vi "CSM - Debug Console - previous.vi"() -> ()   [LabVIEW 2017]
doc: "CSM Debug Console, you can use this tool:\n\n1. Select an existing CSM instance, open the front panel and block diagram.\n2. Scan the API interfaces of existing CSM instances.\n3. Select an API interface, call synchronously or asynchronously, view the return value.\n4. View the overall program's running log."
uses:
  _Support/Typedef/_CSM_List Module Scope.ctl
  Utility/_support/Periodic String Filter Level.ctl
  Utility/Periodic String Filter Setting.ctl
  _Support/Typedef/_CSM_GlobalLog_MSG.ctl
  _Support/Typedef/_CSM_Response Source Message.ctl
  _Support/Typedef/_CSM_GlobalLog_MSG_TYPE.ctl
  1437127e-efa5-494e-aa43-da9d647a7a6f.vi
  6c6a0a0d-4e90-432b-9646-7a8ac0ceadb8.vi
  AdvanceAPI/CSM - Keywords.vi
  AdvanceAPI/CSM - Convert Error to Argument.vi
  _Support/GlobalEvent/GEvt-Generate with Rule Check.vi
  _Support/GlobalEvent/Cache-GEvt Refs.vi
  _Shared/Change Speed Counter.vi
  _Support/ChangeFlag/FlagInstance-GEvt Refs.vi
  _Support/ChangeFlag/ChangeFlag-Read.vi
  _Support/GlobalEvent/LogFilter/LogFilter - Check.vi
  _Support/GlobalEvent/GEvt-Valid Subscribers.vi
  _Support/GlobalEvent/FGV-GlobalEventQueues(lvlibp).vi
  _Support/GlobalEvent/FGV-GlobalEventRef(lvlibp).vi
  _Support/ChangeFlag/ChangeFlagDB.vi
  _Polymophic/Build Interrupt Broadcast Message.vi
  _Polymophic/Build No-Reply Asynchronous Message with Arguments.vi
  _Polymophic/Build Synchronous Message with Arguments.vi
  <vilib>/Utility/config.llb/Close Config Data.vi
  <vilib>/Utility/config.llb/Write Key.vi
  <vilib>/Utility/config.llb/Write Key (Double).vi
  <vilib>/Utility/config.llb/Write Key (I32).vi
  <vilib>/Utility/config.llb/Write Key (String).vi
  _csmHelper/lvcsmFile/Path to lvcsm String.vi
  <vilib>/Utility/config.llb/Remove Key.vi
  <vilib>/Utility/config.llb/Get Key Names.vi
  <vilib>/Utility/Data Type/Get Type Information.vi
  <vilib>/Utility/Data Type/Get Array Information.vi
  <vilib>/Utility/config.llb/Write Key (Boolean).vi
  <vilib>/Utility/config.llb/Open Config Data.vi
  _csmHelper/lvcsmFile/lvcsm File Path.vi
  _csmHelper/lvcsmFile/_Array of VData to VCluster.vi
  <vilib>/Utility/config.llb/Read Key.vi
  <vilib>/Utility/config.llb/Read Key (Double).vi
  <vilib>/Utility/config.llb/Read Key (I32).vi
  _csmHelper/lvcsmFile/lvcsm String to Path.vi
  <vilib>/Utility/config.llb/Read Key (String).vi
  <vilib>/Utility/config.llb/Read Key (Boolean).vi
  _Polymophic/Add State(s) to Queue By BOOL(Element).vi
  _csmHelper/API/Destroy.vi
  _csmHelper/API/Update lvcsm Section in VI Description.vi
  _csmHelper/API/Create From VI Reference.vi
  _Support/GlobalEvent/LogFilter/LogFilter.lvclass
  Communicable State Machine.lvlib
  _csmHelper/API with lvcsm Support/CSM-Helper API with lvcsm Support.lvlib
  _csmHelper/CSM-Helper.lvclass
  _Support/csm-tool-support.lvlib
  _Shared/CSM Shared.lvlib
  _ui/csm-ui-support.lvlib
panel:
  in  "Scope":T1
  in  "Refresh CSMs Button":bool
  in  "CSM":string(combo)
  in  "Write lvcsm in Description":bool
  out "inlvlibp":bool
  in  "RetainWireValues":bool
  in  "Interface-Filter":enum16{"API-Only", "UserDef States", "All"}(ring)
  in  "Toolbar.Exit":bool
  in  "Toolbar.Open FP":bool
  in  "Toolbar.Open BD":bool
  in  "Refresh lvcsm Cache":bool
  in  "History":i32(listbox)
  in  "Refresh API":bool
  in  "MsgString":string(combo)
  in  "Tab(Msg/Status)":enum32{"Message", "Status"}(tab)
  in  "Sync (-@)":bool
  in  "Async (->|)":bool
  in  "Timeout(s)":i32=10 caption="(s)" min=1 max=180 step=1 format="%.0p"
  in  "Broadcast":bool
  in  "Arguments":string
  in  "Revert Safe String":bool=TRUE
  out "Response":string
  in  "Periodic":bool
  in  "Settings":T2={"threashold(#/s)"=0.5, "Check Peroid(s)"=3.0}
  in  "Periodic Info":bool=TRUE
  in  "internal-stop":bool
  out "handling Speed(#/s)":dbl
  in  "Level":T3
  out "LogInQ":i32
  out "State History":string
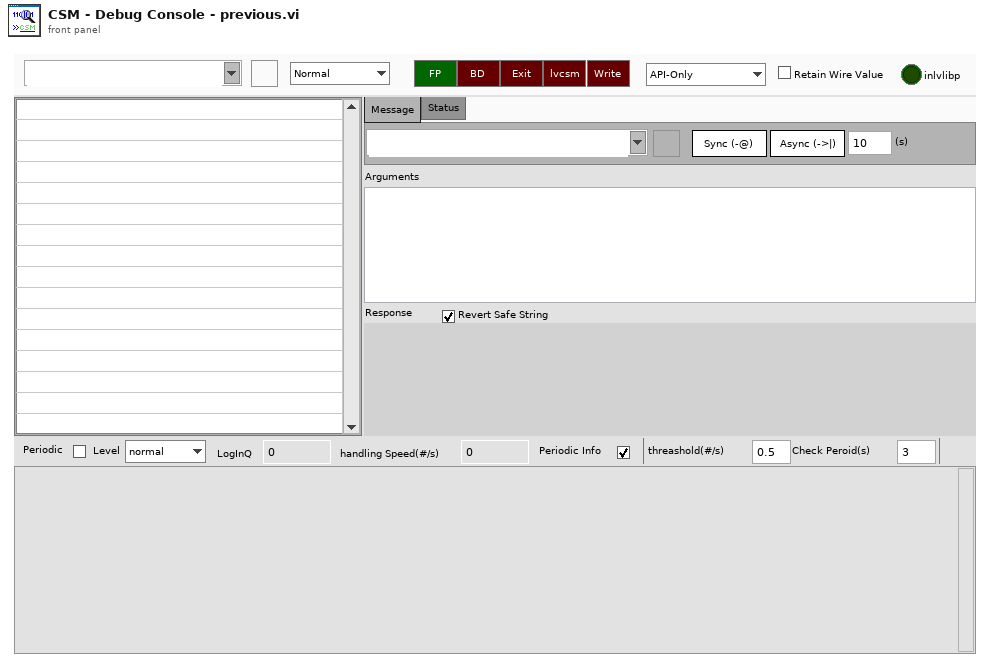
[diagram p1: front panel]
types:
  T1 = typedef "Communicable State Machine.lvlib/_CSM_List Module Scope.ctl" = enum16{"Normal", "System Only", "All"}
  T2 = typedef "Communicable State Machine.lvlib/Periodic String Filter Setting.ctl" = cluster{"threashold(#/s)":dbl, "Check Peroid(s)":dbl}
  T3 = typedef "Communicable State Machine.lvlib/Periodic String Filter Level.ctl" = enum16{"normal", "L1", "L2", "L3", "L4"}
  T4 = enum32{"Invalid", "Standard", "Closed", "Hidden", "Minimized", "Maximized"}
  T5 = enum32{"invalid app kind", "Development System", "Run Time System", "Student Edition", "Embedded LabVIEW", "Evaluation", "Custom"}
  T6 = cluster{"Response Timeout(s)":i32, "History Length":i32, "History":string[], "Periodic Enable":bool, "Periodic threashold(#/s)":dbl, "Periodic Check Peroid(s)":dbl}
  T7 = enum8{"Enabled", "Disabled", "Disabled and Grayed Out"}
  T8 = cluster{"Shift":bool, "Ctrl":bool, "Alt":bool, "Cmd":bool, "Opt":bool}
  T9 = typedef "LVPoint32TypeDef.ctl" = cluster{"Horizontal":i32, "Vertical":i32}
  T10 = cluster{"Core":cluster{"Current VI Reference":refnum<vi>, "Close Panel on Exit?":bool}, "CSM Global Log Event":refnum<user-event>, "MessageList":string[], "Toobar.advance":refnum<vi>[], "CSM Check History":string[], "History Length":i32}
  T11 = cluster{"Current VI Reference":refnum<vi>, "Close Panel on Exit?":bool}
  T12 = cluster{"Periodic threashold(#/s)":dbl, "Periodic Check Peroid(s)":dbl}
  T13 = typedef "Communicable State Machine.lvlib/_CSM_GlobalLog_MSG.ctl" = cluster{"Name (\"\" to Use UUID)":string, "Current State":string, "Arguments":string, "Source Message":T14, "Source Module":string, "Complete(T)/Start(F)":bool, "LogType":T15, "Time Stamp":timestamp}
  T14 = typedef "Communicable State Machine.lvlib/_CSM_Response Source Message.ctl" = cluster{"‘State":string, "’Arguments":string, "’Error":errorcluster}
  T15 = typedef "Communicable State Machine.lvlib/_CSM_GlobalLog_MSG_TYPE.ctl" = enum16{"User Log", "State Change", "Status", "Interrupt", "Register", "Unregister", "Error Log", "Module Created", "Module Destroyed", "Async Message", "No-Rep Async Message", "Sync Message"}
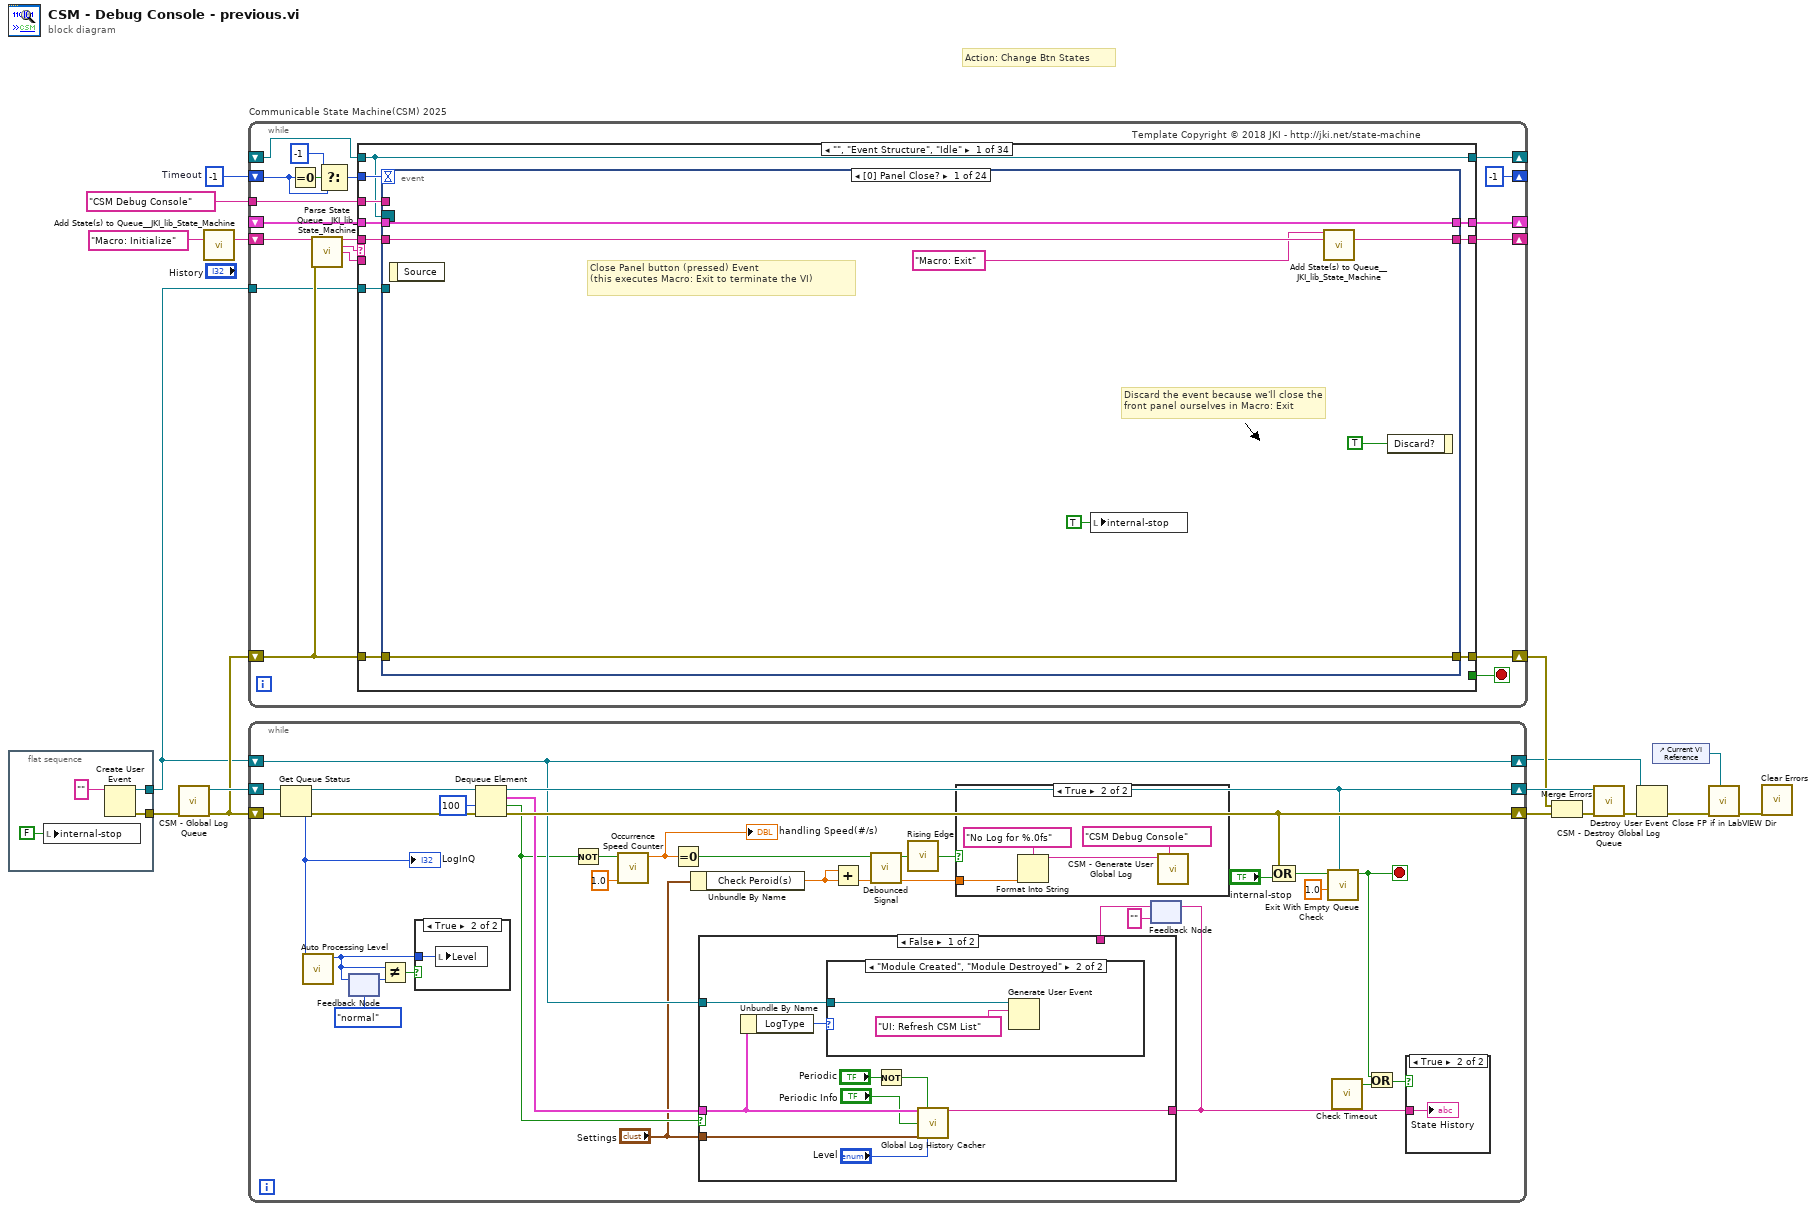
[diagram p0: block diagram]
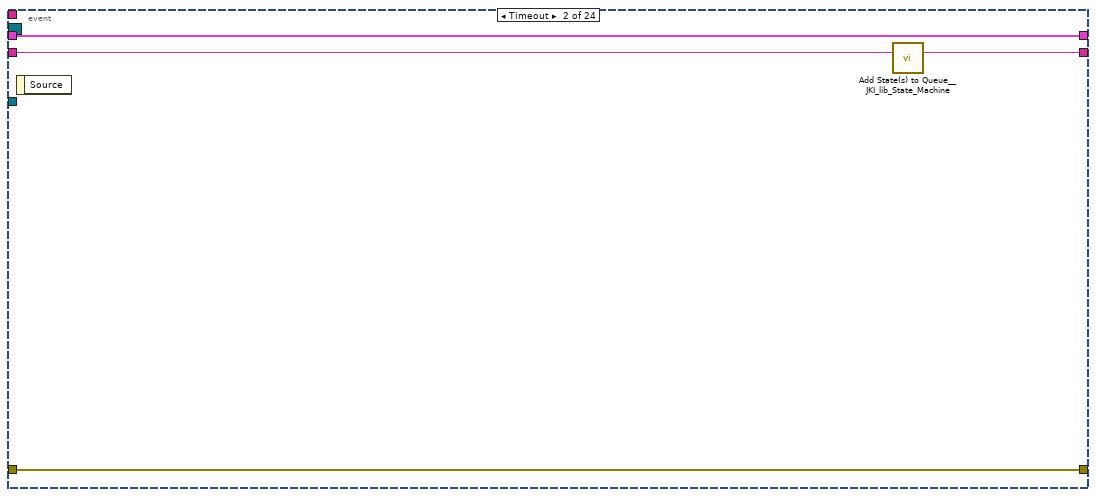
[diagram p7: hidden frame]
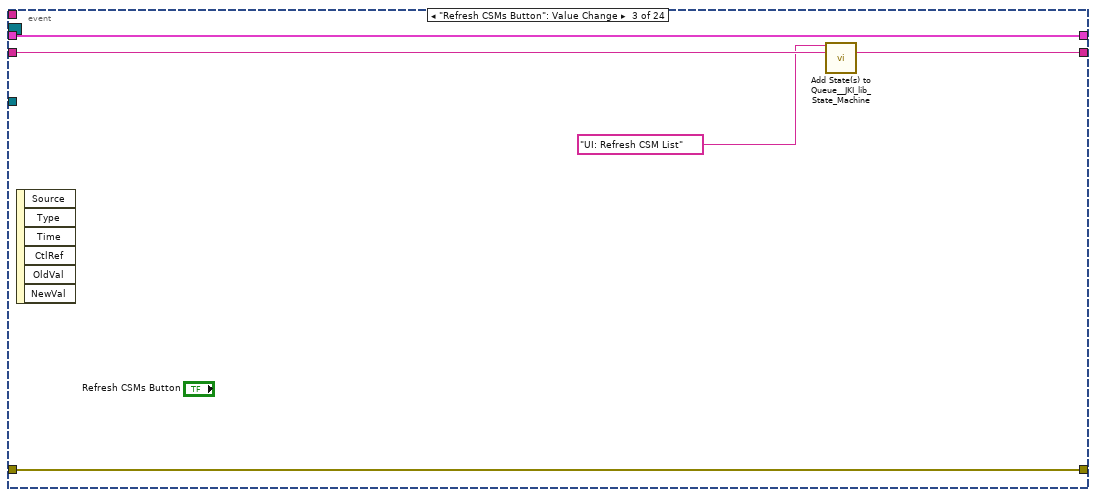
[diagram p8: hidden frame]
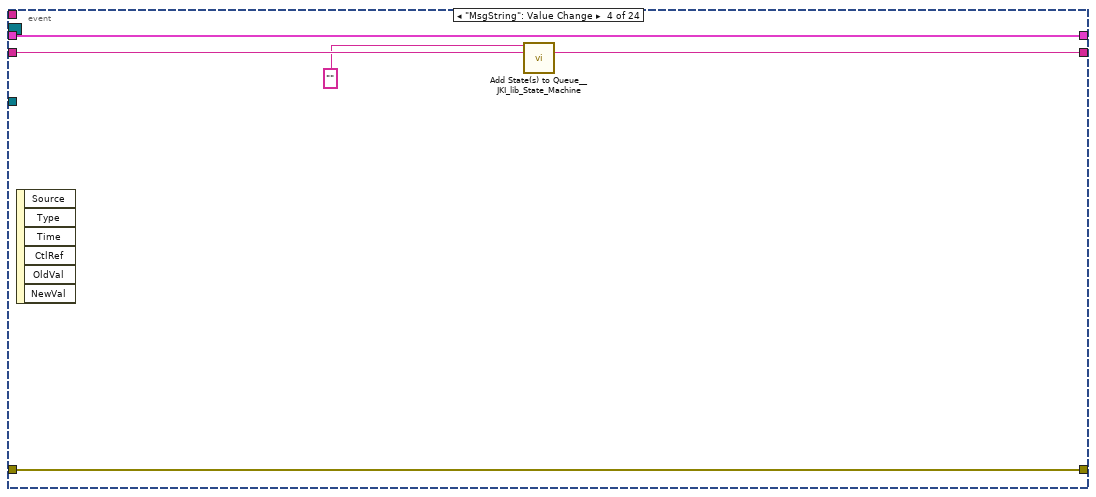
[diagram p9: hidden frame]
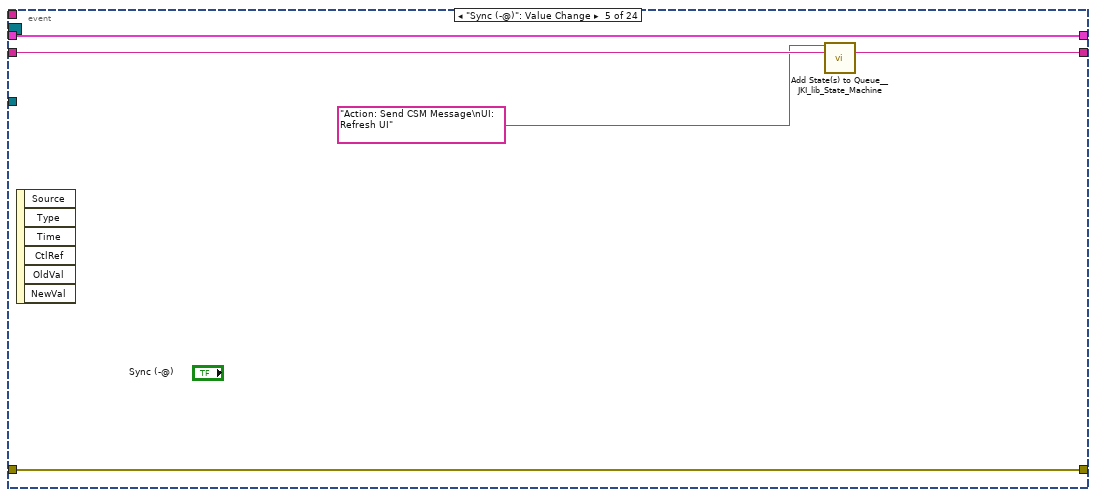
[diagram p10: hidden frame]
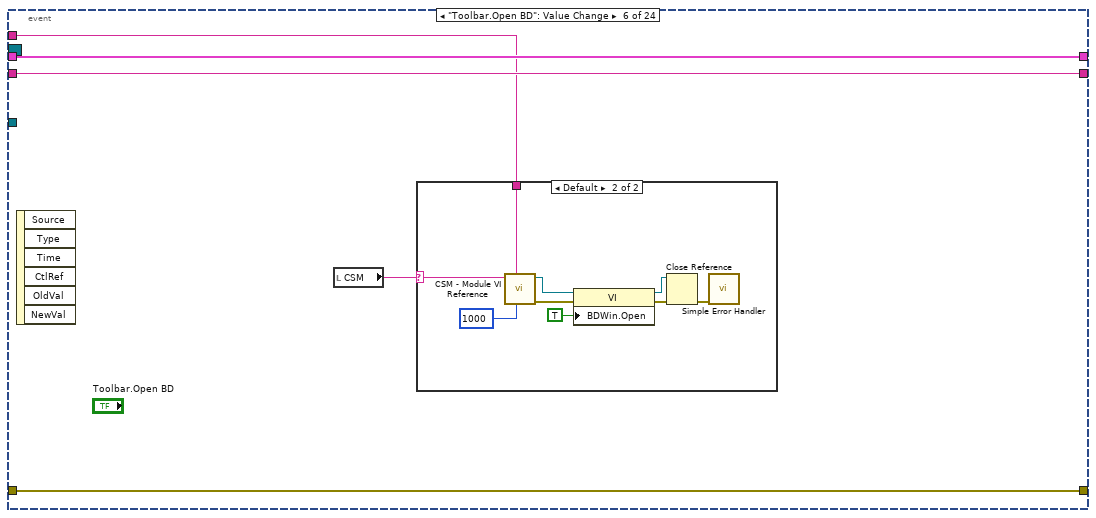
[diagram p11: hidden frame]
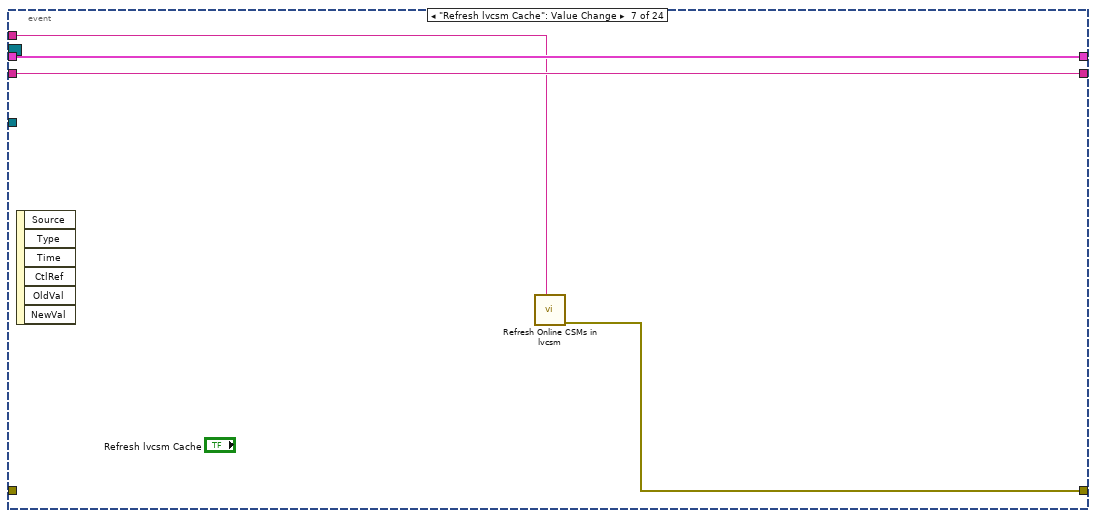
[diagram p13: hidden frame]
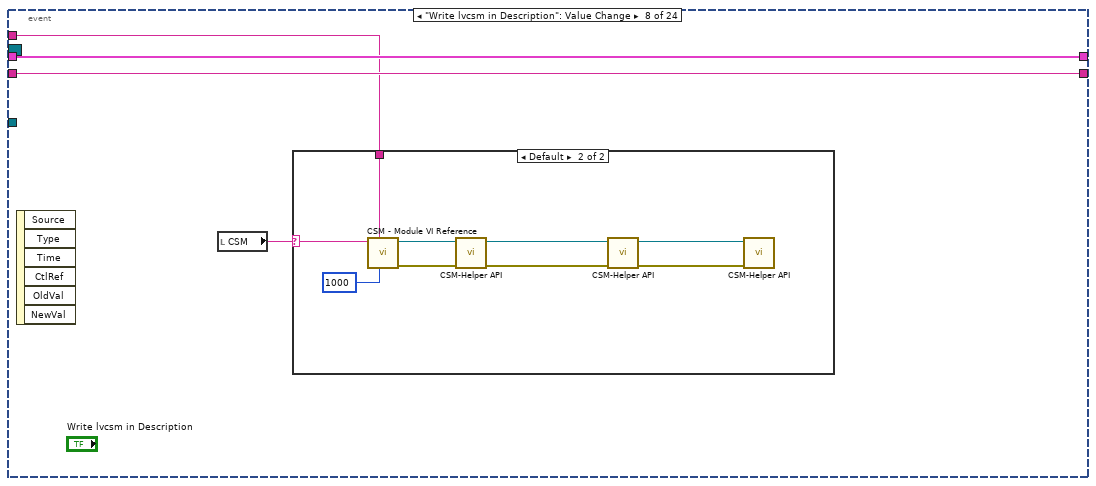
[diagram p14: hidden frame]
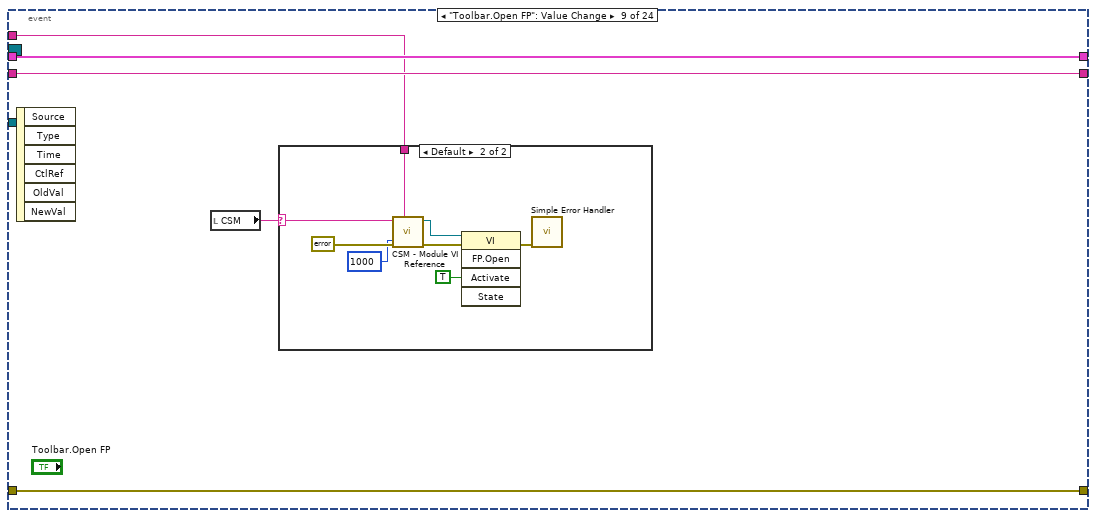
[diagram p16: hidden frame]
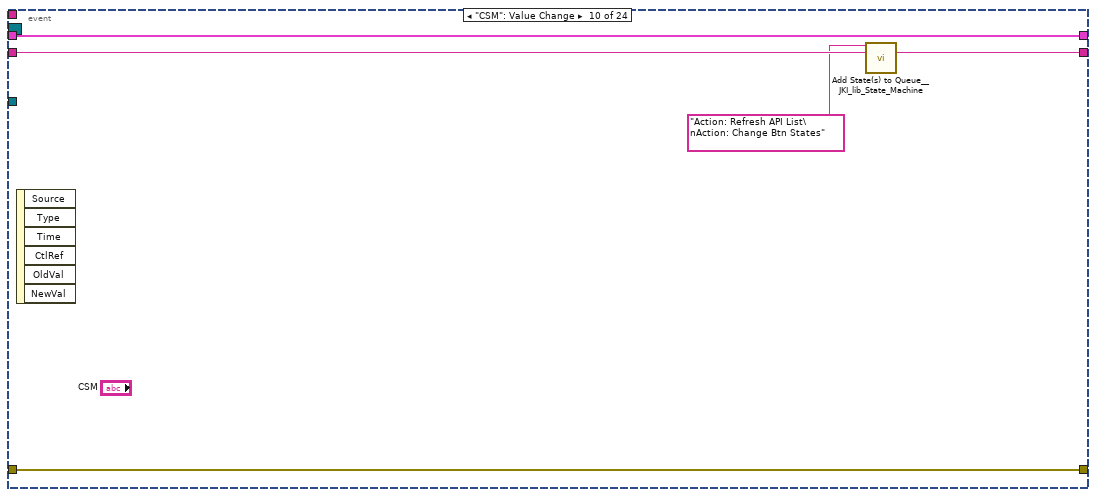
[diagram p18: hidden frame]
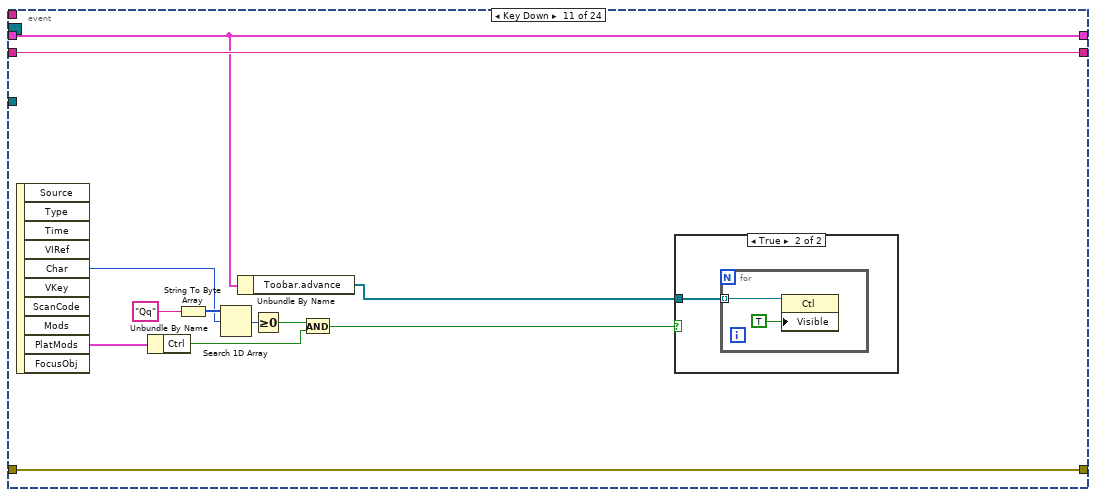
[diagram p19: hidden frame]
diagram:
  w14 = -1  # Timeout
  # "Action: Change Btn States"
  n1 = flat-sequence {
    tunnel: [w21] -> w7
    tunnel: [w19] -> w4
    frame #0 {
      n2 = local write "internal-stop"(FALSE ("internal-stop")) -> ()
      n3 = Create User Event(user event datatype="" ("UserEvent")) -> (user event=w19:refnum<user-event>, error out=w21:errorcluster)  [unwired: 1 in]
    }
  }
  n4 = call "CSM - Global Log Queue.vi"("Error In"=w7) -> ("error out"=w10:errorcluster, "Global Log Queue"=w11:refnum<queue>)  [unwired: 9 in]
  n5 = call <vilib>:"Add State(s) to Queue__JKI_lib_State_Machine.vi"("State(s) in (\"\")"="Macro: Initialize") -> ("States Out"=w16:string)  [unwired: 14 in]
  n6 = while "Communicable State Machine(CSM) 2025" {
    shift-right: [w33] -> _
    shift-left: _ -> [w32]
    shift-right: [w36] -> w8
    shift-left: w10 -> [w31]
    shift-right: [w35] -> _
    shift-left: w16 -> [w37]
    tunnel: "CSM Debug Console" -> [w30]
    shift-right: [-1 ("Timeout")] -> _
    shift-left: w14 -> [w27]
    tunnel: w4 -> [w24]
    shift-right: [w23] -> _
    shift-left: _ -> [w22]
    stop <- w34 stop-if-true
    # "Template Copyright © 2018 JKI - http://jki.net/state-machine"
    n7 = Equal To 0?(x=w27) -> (x = 0?=w29:bool)
    n8 = call <vilib>:"Parse State Queue__JKI_lib_State_Machine.vi"("State Queue"=w37, "Error In (no error)"=w31) -> ("Remaining States"=w39:string, "Current State"=w40:string, "Arguments"=w38:string)  [unwired: 11 in]
    n9 = Select(t=-1 ("Timeout"), s=w29, f=w27) -> (s? t:f=w26:i32)
    n10 = case shown="\"\", \"Event Structure\", \"Idle\"" w40 {
      selector: w40 -> [_ _ w312 _ _ _ _ _ _ _ _ _ _ _ _ _ _ _ _ _ _ _ _ _ _ _ _ _ _ _ _ _ _ _]
      tunnel: w39 -> [w50 w310 w316 w336 w344 w350 w355 w366 w374 w389 w403 w416 w432 w437 w442 w447 w452 w462 w472 w484 w564 w581 w595 w599 w605 w611 w622 w627 w639 w666 w686 w703 w733 w789]
      tunnel: w38 -> [_ _ _ _ _ _ _ _ _ _ _ w412 _ _ _ _ _ _ w467 w478 w563 _ _ _ _ _ _ _ _ _ _ _ _ _]
      tunnel: w32 -> [w48 w307 w314 w329 w341 w348 w352 _ w373 w387 w402 w414 w427 w434 w440 w445 w449 w459 w470 w480 w561 w580 w594 w598 w602 w608 w619 w624 w637 w664 w684 w702 w728 w788]
      tunnel: [w47 w308 w318 w333 errorcluster {"status"=FALSE, "code"=0, "source"=""} ("error out") w347 w353 w363 w375 _ w397 w415 w428 w435 _ w443 w450 w460 w468 w481 w565 w582 w596 w600 w603 w609 w620 w625 w634 w663 w683 w704 w730 w790] -> w36
      tunnel: w31 -> [w46 w308 w317 w333 w340 w347 w353 w363 w375 _ _ w415 w429 w435 _ _ w450 w460 w469 w482 w565 w582 w596 w600 w603 w609 w620 w625 _ _ _ w704 _ w790]
      tunnel: [w49 w309 w315 w335 w343 w349 w354 w365 w374 w389 w403 w416 w431 w436 w441 w446 w451 w461 w471 w483 w564 w581 w595 w599 w604 w610 w621 w626 w638 w665 w685 w703 w733 w789] -> w35
      tunnel: [_ _ _ _ _ TRUE _ _ _ _ _ _ _ _ _ _ _ _ _ _ _ _ _ _ _ _ _ _ _ _ _ _ _ _] -> w34
      tunnel: [w45 w307 w314 w334 w341 w348 w352 w364 w370 w388 w402 w408 w427 w434 w440 w445 w449 w459 w470 w480 w561 w580 w594 w598 w602 w608 w619 w624 w637 w664 w684 w702 w727 w788] -> w33
      tunnel: w26 -> [w44 _ _ _ _ _ _ _ _ _ _ _ _ _ _ _ _ _ _ _ _ _ _ _ _ _ _ _ _ _ _ _ _ _]
      tunnel: w30 -> [w43 _ _ _ w338 _ _ _ _ w384 w398 _ _ _ _ _ _ _ _ _ _ _ _ _ _ _ _ _ _ _ _ w699 w731 w785]
      tunnel: w24 -> [w42 _ _ _ _ _ _ _ _ _ _ _ _ _ w439 _ _ _ _ _ _ _ _ _ _ _ _ _ _ _ _ _ _ _]
      tunnel: [w41 w306 w311 w323 w337 w345 w351 w357 w367 w382 w396 w405 w426 w433 w438 w444 w448 w455 w466 w477 w553 w576 w583 w597 w601 w606 w612 w623 w628 w658 w678 w701 w725 w787] -> w23
      tunnel: w22 -> [w41 w306 w311 w323 w337 w345 w351 w357 w367 w382 w396 w405 w426 w433 _ w444 w448 w455 w466 w477 w553 w576 w583 w597 w601 w606 w612 w623 w628 w658 w678 w701 w725 w787]
      frame "", "Event Structure", "Idle" {
        n11 = event shown="[0] Panel Close?" {
          selector: w41 -> [_ _ _ _ _ _ _ _ _ _ _ _ _ _ _ _ _ _ _ _ _ _ _ _]
          dyn-events: _ -> [_ _ _ _ _ _ _ _ _ _ _ _ _ _ _ _ _ _ _ _ _ _ _ _]
          timeout: w44 -> [_ _ _ _ _ _ _ _ _ _ _ _ _ _ _ _ _ _ _ _ _ _ _ _]
          tunnel: w50 -> [w57 w61 w64 w68 w73 w81 w94 w98 w112 w122 w137 w142 w148 w156 w166 w173 w201 w220 w239 w252 w257 w262 w274 w276]
          tunnel: [w56 w60 w63 w69 w74 w81 w94 w98 w112 w123 w137 w143 w148 w157 w167 w173 w201 w220 w239 w253 w258 w263 w274 w278] -> w49
          tunnel: w48 -> [w54 w58 w65 w70 w75 w80 w93 w97 w111 w124 w126 w144 w146 w163 w168 w172 w199 w218 w237 w254 w259 w264 w272 w279]
          tunnel: [w55 w59 w66 w71 w76 w78 w91 _ w109 w125 w136 w145 w147 w164 _ w171 w200 w219 w238 w255 w260 _ w273 w280] -> w47
          tunnel: w46 -> [w55 w59 w66 w71 w76 w78 _ _ w109 w125 w136 w145 w147 w164 _ w171 w200 w219 w238 w255 w260 _ w273 w280]
          tunnel: [w54 w58 w65 w70 w75 w80 w93 w97 w111 w124 w126 w144 w146 w163 w168 w172 w199 w218 w237 w254 w259 w264 w272 w277] -> w45
          tunnel: w43 -> [_ _ _ _ _ w77 w92 w95 w108 _ _ _ _ _ _ w169 _ w216 _ _ _ _ _ _]
          tunnel: w42 -> [_ _ _ _ _ _ _ _ _ _ _ _ _ _ _ _ _ _ _ _ _ _ _ _]
          event Panel Close? {
            # "Discard the event because we'll close the front panel ourselves in Macro: Exit"
            # "Close Panel button (pressed) Event\n(this executes Macro: Exit to terminate the VI)"
            n12 = event-data() -> ()  [unwired: 1 in, 1 out]
            n13 = local write "internal-stop"(TRUE ("internal-stop")) -> ()
            n14 = call <vilib>:"Add State(s) to Queue__JKI_lib_State_Machine.vi"("State(s) in Front (\"\")"="Macro: Exit", "State(s) in (\"\")"=w57) -> ("States Out"=w56:string)  [unwired: 13 in]
            n15 = event-data("Discard?"=TRUE) -> ()  [unwired: 1 in, 1 out]
          }
          event Timeout {
            n16 = event-data() -> ()  [unwired: 1 in, 1 out]
            n17 = call <vilib>:"Add State(s) to Queue__JKI_lib_State_Machine.vi"("State(s) in (\"\")"=w61) -> ("States Out"=w60:string)  [unwired: 14 in]
          }
          event "Refresh CSMs Button": Value Change {
            n18 = event-data() -> ()  [unwired: 1 in, 6 out]
            n19 = call <vilib>:"Add State(s) to Queue__JKI_lib_State_Machine.vi"("State(s) in Front (\"\")"="UI: Refresh CSM List" ("State(s) in Front (\"\")"), "State(s) in (\"\")"=w64) -> ("States Out"=w63:string)  [unwired: 13 in]
          }
          event "MsgString": Value Change {
            n20 = event-data() -> ()  [unwired: 1 in, 6 out]
            n21 = call <vilib>:"Add State(s) to Queue__JKI_lib_State_Machine.vi"("State(s) in Front (\"\")"="" ("State(s) in Front (\"\")"), "State(s) in (\"\")"=w68) -> ("States Out"=w69:string)  [unwired: 13 in]
          }
          event "Sync (-@)": Value Change {
            n22 = event-data() -> ()  [unwired: 1 in, 6 out]
            n23 = call <vilib>:"Add State(s) to Queue__JKI_lib_State_Machine.vi"("State(s) in Front (\"\")"="Action: Send CSM Message\nUI: Refresh UI" ("State(s) in Front (\"\")"), "State(s) in (\"\")"=w73) -> ("States Out"=w74:string)  [unwired: 13 in]
          }
          event "Toolbar.Open BD": Value Change {
            n24 = event-data() -> ()  [unwired: 1 in, 6 out]
            n25 = local read "CSM"() -> (w79:string)
            n26 = case shown="Default" w79 {
              selector: w79 -> [_ w89]
              tunnel: w77 -> [_ w88]
              frame "" {
              }
              frame Default {
                n27 = call "CSM - Module VI Reference.vi"("Response Timeout (-2 Using Global Settings)"=1000 ("Response Timeout(5000 ms)"), "Current Module (\"\" to Generate an ID)"=w88, "CSM Name"=w89) -> ("error out"=w82:errorcluster, "CSM Module VIRef"=w87:refnum<vi>)  [unwired: 7 in]
                n28 = property class="VI"(reference=w87, error in=w82, "BDWin.Open"=TRUE ("Block Diagram Window:Open")) -> (reference out=w85:refnum<vi>, error out=w84:errorcluster)
                n29 = Close Reference(reference=w85, error in (no error)=w84) -> (error out=w90:errorcluster)
                n30 = call <vilib>:"Simple Error Handler.vi"("error in (no error)"=w90) -> ()  [unwired: 4 in, 5 out]
              }
            }
          }
          event "Refresh lvcsm Cache": Value Change {
            n31 = event-data() -> ()  [unwired: 1 in, 6 out]
            n32 = call "Refresh Online CSMs in lvcsm.vi"("Caller"=w92) -> ("error out"=w91:errorcluster)  [unwired: 9 in, 1 out]
          }
          event "Write lvcsm in Description": Value Change {
            n33 = event-data() -> ()  [unwired: 1 in, 6 out]
            n34 = local read "CSM"() -> (w96:string)
            n35 = case shown="Default" w96 {
              selector: w96 -> [_ w103]
              tunnel: w95 -> [_ w99]
              frame "" {
              }
              frame Default {
                n36 = call "CSM - Module VI Reference.vi"("Response Timeout (-2 Using Global Settings)"=1000 ("Response Timeout(5000 ms)"), "Current Module (\"\" to Generate an ID)"=w99, "CSM Name"=w103) -> ("error out"=w101:errorcluster, "CSM Module VIRef"=w100:refnum<vi>)  [unwired: 7 in]
                n37 = call-poly "CSM-Helper API.vi"("error in (no error)"=w101, "VI"=w100) -> ("error out"=w107:errorcluster, "CSM-Helper.lvclass"=w106:refnum<class "CSM-Helper.lvclass">)  [unwired: 8 in]
                n38 = call-poly "CSM-Helper API.vi"("error in (no error)"=w107, "CSM-Helper in"=w106) -> ("error out"=w105:errorcluster, "CSM-Helper out"=w104:refnum<class "CSM-Helper.lvclass">)  [unwired: 8 in]
                n39 = call-poly "CSM-Helper API.vi"("error in (no error)"=w105, "CSM-Helper in"=w104) -> ()  [unwired: 8 in, 2 out]
              }
            }
          }
          event "Toolbar.Open FP": Value Change {
            n40 = event-data() -> ()  [unwired: 1 in, 6 out]
            n41 = local read "CSM"() -> (w110:string)
            n42 = case shown="Default" w110 {
              selector: w110 -> [_ w120]
              tunnel: w108 -> [_ w118]
              frame "" {
              }
              frame Default {
                n43 = call "CSM - Module VI Reference.vi"("Response Timeout (-2 Using Global Settings)"=1000 ("Response Timeout(5000 ms)"), "Current Module (\"\" to Generate an ID)"=w118, "error in (no error)"=errorcluster {"status"=FALSE, "code"=0, "source"=""}, "CSM Name"=w120) -> ("error out"=w114:errorcluster, "CSM Module VIRef"=w115:refnum<vi>)  [unwired: 6 in]
                n44 = invoke on="Invoke Node" class="VI" method="FP.Open"(reference=w115, error in=w114, "Activate"=TRUE ("Activate?")) -> (error out=w119:errorcluster)  [unwired: 2 in, 4 out]
                n45 = call <vilib>:"Simple Error Handler.vi"("error in (no error)"=w119) -> ()  [unwired: 4 in, 5 out]
              }
            }
          }
          event "CSM": Value Change {
            n46 = event-data() -> ()  [unwired: 1 in, 6 out]
            n47 = call <vilib>:"Add State(s) to Queue__JKI_lib_State_Machine.vi"("State(s) in Front (\"\")"="Action: Refresh API List\nAction: Change Btn States" ("State(s) in Front (\"\")"), "State(s) in (\"\")"=w122) -> ("States Out"=w123:string)  [unwired: 13 in]
          }
          event Key Down {
            n48 = event-data() -> ("Char"=w127:i16, "PlatMods"=w128:T8)  [unwired: 1 in, 8 out]
            n49 = Unbundle By Name(w128) -> ("Ctrl"=w131:bool)
            n50 = String To Byte Array(string="Qq") -> (unsigned byte array=w133:u8[])
            n51 = Search 1D Array(1D array=w133, element=w127) -> (index of element=w134:i32)  [unwired: 1 in]
            n52 = Unbundle By Name(w126) -> ("Toobar.advance"=w129:refnum<vi>[])
            n53 = Greater Or Equal To 0?(x=w134) -> (x >= 0?=w135:bool)
            n54 = And(x=w135, y=w131) -> (x .and. y?=w130:bool)
            n55 = case shown="True" w130 {
              tunnel: w129 -> [_ w138]
              frame False {
              }
              frame True {
                n56 = for {
                  tunnel: w138 -> [w140] mode=indexing
                  n57 = property class="Ctl"(reference=w140, "Visible"=TRUE) -> ()  [unwired: 1 in, 2 out]
                }
              }
            }
          }
          event "Async (->|)": Value Change {
            n58 = event-data() -> ()  [unwired: 1 in, 6 out]
            n59 = call <vilib>:"Add State(s) to Queue__JKI_lib_State_Machine.vi"("State(s) in Front (\"\")"="Action: Post CSM Message" ("State(s) in Front (\"\")"), "State(s) in (\"\")"=w142) -> ("States Out"=w143:string)  [unwired: 13 in]
          }
          event "Timeout(s)": Value Change {
            n60 = event-data() -> ()  [unwired: 1 in, 6 out]
          }
          event "History": Double Click {
            n61 = event-data() -> ("CtlRef"=w162:refnum<vi>, "Coords"=w150:T9)  [unwired: 1 in]
            n62 = invoke class="LstBox (strict)" method="Point To Row"(reference=w162, "Point"=w150) -> (reference out=w161:refnum<vi>, error out=w160:errorcluster, "Row"=w149:i32)  [unwired: 5 in, 4 out]
            n63 = property class="LstBox (strict)"(reference=w161, error in=w160) -> ("Item Names"=w158:string[])  [unwired: 2 out]
            n64 = Array Size(array=w158) -> (size(s)=w159:i32)
            n65 = Less?(x=w149, y=w159) -> (x < y?=w155:bool)
            n66 = Index Array(array=w158, index=w149) -> (element=w154:string)
            n67 = call "CSM - Make String Arguments Safe.vi"("Argument String"=w154) -> ("Safe Argument String"=w153:string)  [unwired: 8 in]
            n68 = call <vilib>:"Build State String with Arguments__JKI_lib_State_Machine.vi"("Arguments (\"\")"=w153, "State"="UI: Autoset Arguments") -> ("State with Arguments"=w151:string)  [unwired: 4 in]
            n69 = call-poly "Add State(s) to Queue By BOOL++.vi"("TRUE (\"\")"=w151, "Condition"=w155, "State Queue (\"\")"=w156) -> ("Remaining States"=w157:string)  [unwired: 8 in]
          }
          event "Refresh API": Value Change {
            n70 = event-data() -> ()  [unwired: 1 in, 6 out]
            n71 = call <vilib>:"Add State(s) to Queue__JKI_lib_State_Machine.vi"("State(s) in Front (\"\")"="Action: Refresh API List" ("State(s) in Front (\"\")"), "State(s) in (\"\")"=w166) -> ("States Out"=w167:string)  [unwired: 13 in]
          }
          event "Toolbar.Exit": Value Change {
            n72 = event-data() -> ()  [unwired: 1 in, 6 out]
            n73 = local read "CSM"() -> (w170:string)
            n74 = case shown="Default" w170 {
              selector: w170 -> [_ w176]
              tunnel: w169 -> [_ w179]
              frame "" {
              }
              frame Default {
                n75 = Build Array(w176) -> (w175:string[])
                n76 = call "CSM - Build Exit Messages of CSMs.vi"("CSMs"=w175) -> ("States"=w177:string)  [unwired: 14 in]
                n77 = call "CSM - Run Script.vi"("CSM Scripts"=w177, "Current Module (\"\" to Generate an ID)"=w179, "Continue If Error? (F)"=TRUE) -> ("error out"=w178:errorcluster)  [unwired: 10 in, 2 out]
                n78 = call <vilib>:"Simple Error Handler.vi"("error in (no error)"=w178) -> ()  [unwired: 4 in, 5 out]
              }
            }
          }
          event "State History": Shortcut Menu Activation? {
            n79 = event-data() -> ("CtlRef"=w197:refnum<vi>, "MenuRef"=w198:refnum<k9>, "Coords"=w196:T9)  [unwired: 1 in, 4 out]
            n80 = invoke class="Str" method="ByteOffFromPt"(reference=w197, "Point"=w196) -> (reference out=w195:refnum<vi>, error out=w193:errorcluster, "ByteOffFromPt"=w194:i32)  [unwired: 2 in, 1 out]
            n81 = property class="Str"(reference=w195, error in=w193) -> (error out=w185:errorcluster, "Text.Text"=w191:string)  [unwired: 1 out]
            n82 = String Subset(string=w191, length (rest)=w194) -> (substring=w192:string)  [unwired: 1 in]
            n83 = call "CSM - Break Down Multiple States String.vi"("States"=w191) -> ("Multiple States"=w190:string[])  [unwired: 10 in]
            n84 = call "CSM - Break Down Multiple States String.vi"("States"=w192) -> ("Multiple States"=w189:string[])  [unwired: 10 in]
            n85 = Array Size(array=w189) -> (size(s)=w188:i32)
            n86 = Decrement(x=w188) -> (x-1=w187:i32)
            n87 = Index Array(array=w190, index=w187) -> (element=w186:string)
            n88 = call "Trim Single-line Text.vi"("single-line text"=w186) -> ("trimed text"=w184:string)  [unwired: 2 in]
            n89 = call "_parse Log Line.vi"("String"=w184) -> ("LogType"=w182:string, "State"=w180:string, "CSM"=w181:string)  [unwired: 8 in]
            n90 = case shown="\"State Change\"" w182 {
              tunnel: w198 -> [w211 _]
              tunnel: w184 -> [_ _]
              tunnel: w185 -> [w209 _]
              tunnel: [_ TRUE] -> w183
              tunnel: w181 -> [w207 _]
              tunnel: w180 -> [w206 _]
              frame "State Change" {
                n91 = Format Into String(format string="\"%s@%s\"", w206, w207) -> (resulting string=w202:string)  [unwired: 2 in, 1 out]
                n92 = Concatenate Strings("Go To " ("format string"), w202) -> (w205:string)
                n93 = Concatenate Strings("GO_TO_STATE_" ("item tags"), w202) -> (w203:string)
                n94 = Insert Menu Items(6:w209, 7:w203, 8:w205, 9:w211) -> ()  [unwired: 2 in, 3 out]
              }
              frame Default {
              }
            }
            n95 = event-data("Discard?"=w183) -> ()  [unwired: 1 in, 1 out]
          }
          event "RetainWireValues": Value Change {
            n96 = event-data() -> ("CtlRef"=w214:refnum<vi>, "OldVal"=w213:bool, "NewVal"=w215:bool)  [unwired: 1 in, 3 out]
            n97 = local read "CSM"() -> (w217:string)
            n98 = case shown="Default" w217 {
              selector: w217 -> [_ w226]
              tunnel: w216 -> [_ w225]
              tunnel: w215 -> [_ w224]
              tunnel: w214 -> [_ w222]
              tunnel: w213 -> [_ w221]
              frame "" {
              }
              frame Default {
                n99 = call "CSM - Module VI Reference.vi"("Current Module (\"\" to Generate an ID)"=w225, "CSM Name"=w226) -> ("error out"=w228:errorcluster, "CSM Module VIRef"=w227:refnum<vi>)  [unwired: 8 in]
                n100 = property class="VI"(reference=w227, error in=w228, "Exec.PostExecutionProbes"=w224) -> (error out=w223:errorcluster)  [unwired: 1 out]
                n101 = case shown="Error" w223 {
                  selector: w223 -> [_ w229]
                  tunnel: w222 -> [_ w231]
                  tunnel: w221 -> [_ w230]
                  frame No Error {
                  }
                  frame Error {
                    n102 = call <vilib>:"Simple Error Handler.vi"("error in (no error)"=w229) -> ()  [unwired: 4 in, 5 out]
                    n103 = property class="Bool (strict)"(reference=w231, "Value"=w230) -> ()  [unwired: 1 in, 2 out]
                  }
                }
              }
            }
          }
          event "State History": Shortcut Menu Selection (User) {
            n104 = event-data() -> ("ItemTag"=w233:string)  [unwired: 1 in, 7 out]
            n105 = Match Pattern(string=w233, regular expression="^GO_TO_STATE") -> (after substring=w232:string, offset past match=w235:i32)  [unwired: 1 in, 2 out]
            n106 = Greater Or Equal To 0?(x=w235) -> (x >= 0?=w234:bool)
            n107 = case shown="True" w234 {
              tunnel: w232 -> [_ w250]
              frame False {
              }
              frame True {
                n108 = Match Pattern(string=w250, regular expression="\"") -> (after substring=w247:string)  [unwired: 1 in, 3 out]
                n109 = Match Pattern(string=w247, regular expression="\"") -> (before substring=w246:string)  [unwired: 1 in, 3 out]
                n110 = Match Pattern(string=w246, regular expression="@") -> (before substring=w244:string, after substring=w243:string)  [unwired: 1 in, 2 out]
                n111 = call "Trim Single-line Text.vi"("single-line text"=w244) -> ("trimed text"=w242:string)  [unwired: 2 in]
                n112 = call "Trim Single-line Text.vi"("single-line text"=w243) -> ("trimed text"=w241:string)  [unwired: 2 in]
                n113 = call "Jump to CSM State.vi"("State"=w242, "Name"=w241) -> ("error out"=w240:errorcluster)  [unwired: 9 in]
                n114 = call <vilib>:"Simple Error Handler.vi"("error in (no error)"=w240) -> ()  [unwired: 4 in, 5 out]
              }
            }
          }
          event User Event {
            n115 = event-data() -> ("UserEvent"=w251:string)  [unwired: 1 in, 4 out]
            n116 = call <vilib>:"Add State(s) to Queue__JKI_lib_State_Machine.vi"("State(s) in Front (\"\")"=w251, "State(s) in (\"\")"=w252) -> ("States Out"=w253:string)  [unwired: 13 in]
          }
          event "Broadcast": Value Change {
            n117 = event-data() -> ()  [unwired: 1 in, 6 out]
            n118 = call <vilib>:"Add State(s) to Queue__JKI_lib_State_Machine.vi"("State(s) in Front (\"\")"="Action: Broadcast Status\nUI: Refresh UI" ("State(s) in Front (\"\")"), "State(s) in (\"\")"=w257) -> ("States Out"=w258:string)  [unwired: 13 in]
          }
          event "Tab(Msg/Status)": Value Change {
            n119 = event-data() -> ()  [unwired: 1 in, 6 out]
            n120 = call <vilib>:"Add State(s) to Queue__JKI_lib_State_Machine.vi"("State(s) in Front (\"\")"="Action: Refresh API List" ("State(s) in Front (\"\")"), "State(s) in (\"\")"=w262) -> ("States Out"=w263:string)  [unwired: 13 in]
          }
          event "History": Shortcut Menu Activation? {
            n121 = event-data() -> ("MenuRef"=w271:refnum<k9>)  [unwired: 1 in, 6 out]
            n122 = Index Array(array=string[][] [["Set History Length", "SET_HISTORY_LEN_MENU"], ["APP_SEPARATOR", "APP_SEPARATOR"], ["Clear All...", "CLEAR_HISOTRY_MENU"]] ("item names"), index (col) #1=0 ("index (row)"), index (col) #2=1 ("index (row)")) -> (element #1=w269:string[], element #2=w267:string[])  [unwired: 2 in]
            n123 = Insert Menu Items(7:w267, 8:w269, 9:w271) -> ()  [unwired: 3 in, 3 out]
            n124 = event-data("Discard?"=FALSE) -> ()  [unwired: 1 in, 1 out]
          }
          event "History": Shortcut Menu Selection (User) {
            n125 = event-data() -> ("ItemTag"=w275:string)  [unwired: 1 in, 7 out]
            n126 = case shown="\"SET_HISTORY_LEN_MENU\"" w275 {
              tunnel: w279 -> [w282 w289 w298]
              tunnel: [w281 w288 w297] -> w278
              tunnel: [w282 w287 w296] -> w277
              tunnel: w276 -> [w281 w285 w297]
              frame Default {
              }
              frame "CLEAR_HISOTRY_MENU" {
                n127 = Two Button Dialog(message="Clear Command History List?") -> (T button?=w283:bool)  [unwired: 2 in]
                n128 = case shown="True" w283 {
                  tunnel: w289 -> [w290 w293]
                  tunnel: [w290 w292] -> w287
                  frame False {
                  }
                  frame True {
                    n129 = Bundle By Name(cluster=w293, "MessageList"=string[] []) -> (w292:T10)
                  }
                }
                n130 = call-poly "Add State(s) to Queue By BOOL++.vi"("TRUE (\"\")"="UI: Refresh History List" ("State(s) in Front (\"\")"), "Condition"=w283, "State Queue (\"\")"=w285) -> ("Remaining States"=w288:string)  [unwired: 8 in]
              }
              frame "SET_HISTORY_LEN_MENU" {
                n131 = call "Change CSM Debugging History Length"() -> ("History Length"=w295:dbl, "OK"=w294:bool)  [unwired: 17 in, 1 out]
                n132 = case shown="True" w294 {
                  tunnel: w298 -> [w299 w305]
                  tunnel: [w299 w304] -> w296
                  tunnel: w295 -> [_ w302]
                  frame False {
                  }
                  frame True {
                    n133 = To Long Integer(number=w302) -> (32bit integer=w300:i32)
                    n134 = Max & Min(x=w300, y=50) -> (max(x,y)=w303:i32)  [unwired: 1 out]
                    n135 = Bundle By Name(cluster=w305, "History Length"=w303) -> (w304:T10)
                  }
                }
              }
            }
          }
        }
      }
      frame "---------- Core ----------" {
        # "Do not put any code in this frame.\n(it is a separator no-op)"
        n136 = call <vilib>:"Add State(s) to Queue__JKI_lib_State_Machine.vi"("State(s) in (\"\")"=w310) -> ("States Out"=w309:string)  [unwired: 14 in]
      }
      frame Default {
        w321 = 42 items=["No error", "Argument error", "Memory is full", "Out of zone", "End of file", "File already open", "Generic file I/O error", "File not found", "File permission error", "Disk is full", "Duplicate path", "Too many files open", "System feature not enabled", "Resource file not found", "Cannot add resource", "Resource not found", "Image not found", "Image memory error", "Pen does not exist", "Config type invalid", "Config token not found", "Config parse error", "Config memory error", "Bad external code format", "Bad external code offset", "External code not present", "Null window", "Destroy window error", "Null menu", "Print aborted", "Bad print record", "Print driver error", "Windows error during printing", "Memory error during printing", "Print dialog error", "Generic print error", "Invalid device refnum", "Device not found", "Device parameter error", "Device unit error", "Cannot open device", "Device call aborted", "Generic error", "Cancelled by user", "Object ID too low", "Object ID too high", "Object not in heap", "Unknown heap", "Unknown object (invalid DefProc)", "Unknown object (DefProc not in table)", "Message out of range", "Invalid (null) method", "Unknown message", "Manager call not supported", "Bad address", "Network operation in progress", "Network operation timed out", "Connection is busy", "Network attribute not supported", "Network error", "Address in use", "System out of memory", "Connection aborted", "Connection refused", "Not connected", "Already connected", "Connection closed", "Initialization error (interapplication manager)", "Bad occurrence", "Wait on unbound occurrence handler", "Occurrence queue overflow", "Datalog type conflict", "Unused", "Unrecognized type (interapplication manager)", "Memory corrupt", "Failed to make temporary DLL", "Old CIN version", "Drag socket not found", "Failed to load drop-object", "Failed to register OLE object", "Failed to release OLE object", "Format specifier type mismatch", "Unknown format specifier", "Too few format specifiers", "Too many format specifiers", "Scan failed", "Newer CIN version", "Error converting to variant", "Runtime menu error", "Password tampered", "Variant attribute not found", "Incompatible variant data type", "Event data is not available", "Event Store is not present", "Occurrence is not found", "Event Queue is not created", "Event info is not available", "Refnum passed is NULL", "Error retrieving Class GUID", "Error retrieving CoClass GUID", "Error retrieving TypeLib GUID.", "Bad built application magic bytes.", "Specific driver is different from the specific driver associated with the Logical Name.", "There is no session opened to the class driver.", "Max Error", "MAX - Error with config objects", "MAX - Error loading configuration", "MAX - Group not supported"]
        # "Current State"
        # "Do not delete, rename, or modify this frame.\n(this is used to capture unhandled states and typos)"
        # "Handle mistyped state name (developer tool)"
        n137 = Format Into String(format string="Software Exception: Unhandled State \"%s\"." ("message"), error in=w317, w312) -> (resulting string=w320:string, error out=w319:errorcluster)  [unwired: 1 in]
        n138 = call <vilib>:"Error Cluster From Error Code.vi"("show call chain? (False)"=TRUE, "error in (no error)"=w319, "error message (\"\")"=w320, "error code (0)"=w321) -> ("error out"=w318:errorcluster)  [unwired: 5 in]
        n139 = call <vilib>:"Add State(s) to Queue__JKI_lib_State_Machine.vi"("State(s) in (\"\")"=w316) -> ("States Out"=w315:string)  [unwired: 14 in]
      }
      frame "Initialize Core Data" {
        # "Do not delete, rename, or modify this frame.\n(this is used to determine panel behavior on exit)"
        # "originally closed?"
        # "exe?"
        # "If panel starts closed or is an EXE, then close it when we exit"
        n140 = property class="VI"() -> ("FP.State"=w326:T4)  [unwired: 2 in, 2 out]
        n141 = property class="App"() -> ("App.Kind"=w332:T5)  [unwired: 2 in, 2 out]
        n142 = control-ref of="Current VI Reference"() -> (w327:refnum<vi>)
        n143 = Equal?(x=w326, y=T4."Closed" ("Front Panel Window:State")) -> (x = y?=w324:bool)
        n144 = Equal?(x=w332, y=T5."Run Time System" ("Application:Kind")) -> (x = y?=w330:bool)
        n145 = Or(x=w324, y=w330) -> (x .or. y?=w328:bool)
        n146 = Bundle By Name(cluster=w329, "Core.Current VI Reference"=w327, "Core.Close Panel on Exit?"=w328) -> (w334:T10)
        n147 = call <vilib>:"Add State(s) to Queue__JKI_lib_State_Machine.vi"("State(s) in (\"\")"=w336) -> ("States Out"=w335:string)  [unwired: 14 in]
      }
      frame "Error Handler" {
        # "Unhandled Error -- Display it"
        # "Handle any errors here.\nYou can also output any states to clean-up after errors occur"
        # "Clear error"
        n148 = call "CSM - Global Log Error Handler.vi"("Place (\"\" to Use VI's Name)"=w338, "Error In"=w340) -> ()  [unwired: 9 in, 1 out]
        n149 = call <vilib>:"Add State(s) to Queue__JKI_lib_State_Machine.vi"("State(s) in Front (\"\")"="/* Post Error States", "State(s) in (\"\")"=w344) -> ("States Out"=w343:string)  [unwired: 13 in]
      }
      frame "Exit" {
        # "Do not put any code in this frame.\n(No errors that occur here will be handled.)"
        n150 = call <vilib>:"Add State(s) to Queue__JKI_lib_State_Machine.vi"("State(s) in (\"\")"=w350) -> ("States Out"=w349:string)  [unwired: 14 in]
      }
      frame "---------- Data ----------" {
        # "Do not put any code in this frame.\n(It is a separator no-op. You can make a copy of this frame to create a new Data frame)"
        n151 = call <vilib>:"Add State(s) to Queue__JKI_lib_State_Machine.vi"("State(s) in (\"\")"=w355) -> ("States Out"=w354:string)  [unwired: 14 in]
      }
      frame "Data: Initialize" {
        w356 = 50  # History Length
        w358 = string[] []  # CSM Check History
        w359 = refnum<vi>[] []  # Toobar.advance
        w360 = string[] []  # MessageList
        w361 = refnum<user-event> refnum  # CSM Global Log Event
        w362 = T11 {"Current VI Reference"=refnum, "Close Panel on Exit?"=FALSE}  # Core
        # "Initialize the shift-register data, here.\n(data names are defined by what you wire into the bundle function)"
        n152 = Bundle("Core"=w362, "CSM Global Log Event"=w361, "MessageList"=w360, "Toobar.advance"=w359, "CSM Check History"=w358, "History Length"=w356) -> (w364:T10)  [unwired: 1 in]
        n153 = call <vilib>:"Add State(s) to Queue__JKI_lib_State_Machine.vi"("State(s) in (\"\")"=w366) -> ("States Out"=w365:string)  [unwired: 14 in]
      }
      frame "Data: Initialize References" {
        n154 = control-ref of="Toolbar.Open FP"() -> (w372:refnum<vi>)
        n155 = control-ref of="Toolbar.Open BD"() -> (w371:refnum<vi>)
        n156 = control-ref of="Refresh lvcsm Cache"() -> (w368:refnum<vi>)
        n157 = Build Array(w372, w371, w368) -> (w369:refnum<vi>[])
        n158 = Bundle By Name(cluster=w373, "Toobar.advance"=w369) -> (w370:T10)
      }
      frame "Data: Load Arguments Config File" {
        n159 = call "lvcsm Read Cluster.vim"("Section"=w384, "Default Prototype"=T6 {"Response Timeout(s)"=30, "History Length"=50, "History"=[], "Periodic Enable"=TRUE, "Periodic threashold(#/s)"=0.5, "Periodic Check Peroid(s)"=3.0}) -> ("Cluster (Dup)"=w386:T6)  [unwired: 8 in, 1 out]
        n160 = Unbundle By Name(w386) -> ("Response Timeout(s)"=w385:i32, "History Length"=w376:i32, "History"=w383:string[], "Periodic Enable"=w381:bool, "Periodic threashold(#/s)"=w380:dbl, "Periodic Check Peroid(s)"=w377:dbl)
        n161 = Bundle("Periodic threashold(#/s)"=w380, "Periodic Check Peroid(s)"=w377) -> (w378:T12)  [unwired: 1 in]
        n162 = local write "Settings"(w378) -> ()
        n163 = local write "Periodic"(w381) -> ()
        n164 = local write "Timeout(s)"(w385) -> ()
        n165 = Bundle By Name(cluster=w387, "History Length"=w376, "MessageList"=w383) -> (w388:T10)
      }
      frame "Data: Save Arguments Config File" {
        n166 = Unbundle By Name(w402) -> ("MessageList"=w399:string[], "History Length"=w390:i32)
        n167 = local read "Timeout(s)"() -> (w400:i32)
        n168 = local read "Settings"() -> (w393:T2)
        n169 = Unbundle By Name(w393) -> ("threashold(#/s)"=w392:dbl, "Check Peroid(s)"=w391:dbl)
        n170 = local read "Periodic"() -> (w394:bool)
        n171 = Bundle By Name(cluster=T6 {"Response Timeout(s)"=30, "History Length"=50, "History"=[], "Periodic Enable"=TRUE, "Periodic threashold(#/s)"=0.5, "Periodic Check Peroid(s)"=3.0}, "History"=w399, "Response Timeout(s)"=w400, "History Length"=w390, "Periodic Enable"=w394, "Periodic threashold(#/s)"=w392, "Periodic Check Peroid(s)"=w391) -> (w401:T6)
        n172 = call "lvcsm Write Cluster.vim"("Section"=w398, "Configuration"=w401) -> ("error out"=w397:errorcluster)  [unwired: 9 in]
      }
      frame "Data: Update Message List" {
        n173 = Unbundle By Name(w414) -> ("MessageList"=w413:string[], "History Length"=w404:i32)
        n174 = call "CSM - Revert Arguments-Safe String.vi"("Safe Argument String"=w412) -> ("Origin Argument String"=w411:string)  [unwired: 8 in]
        n175 = Build Array (concatenate)(w411, w413) -> (w410:string[])
        n176 = for {
          tunnel: w410 -> [w420] mode=indexing
          shift-right: [w419] -> w406
          shift-left: string[] [] -> [w418]
          i -> [w417]
          n177 = Search 1D Array(1D array=w418, element=w420) -> (index of element=w421:i32)  [unwired: 1 in]
          n178 = case shown="-1" w421 {
            tunnel: w420 -> [_ w425]
            tunnel: [w422 w423] -> w419
            tunnel: w418 -> [w422 w424]
            tunnel: w417 -> [_ _]
            frame Default {
            }
            frame -1 {
              n179 = Build Array (concatenate)(w424, w425) -> (w423:string[])
            }
          }
        }
        n180 = Array Subset(array=w406, length=w404) -> (w407:string[])  [unwired: 1 in]
        n181 = Bundle By Name(cluster=w414, "MessageList"=w407) -> (w408:T10)
      }
      frame "Data: Cleanup" {
        # "Cleanup any data and references, here.\n(this is called automatically, by the Macro: Exit)"
        n182 = Unbundle By Name(w427) -> ("Core.Current VI Reference"=w430:refnum<vi>)
        n183 = Close Reference(reference=w430, error in (no error)=w429) -> (error out=w428:errorcluster)
        n184 = call <vilib>:"Add State(s) to Queue__JKI_lib_State_Machine.vi"("State(s) in (\"\")"=w432) -> ("States Out"=w431:string)  [unwired: 14 in]
      }
      frame "---------- Events ----------" {
        # "Do not put any code in this frame.\n(It is a separator no-op. You can make a copy of this frame to create a new UI frame)"
        n185 = call <vilib>:"Add State(s) to Queue__JKI_lib_State_Machine.vi"("State(s) in (\"\")"=w437) -> ("States Out"=w436:string)  [unwired: 14 in]
      }
      frame "Events: Register" {
        # "Do not put any code in this frame.\n(It is a separator no-op. You can make a copy of this frame to create a new UI frame)"
        n186 = register-events(w439) -> (reference out=w438:refnum<event-registration>)  [unwired: 2 in, 1 out]
        n187 = call <vilib>:"Add State(s) to Queue__JKI_lib_State_Machine.vi"("State(s) in (\"\")"=w442) -> ("States Out"=w441:string)  [unwired: 14 in]
      }
      frame "Events: Unregister" {
        # "Do not put any code in this frame.\n(It is a separator no-op. You can make a copy of this frame to create a new UI frame)"
        n188 = Unregister For Events(event registration refnum=w444) -> (error out=w443:errorcluster)  [unwired: 1 in]
        n189 = call <vilib>:"Add State(s) to Queue__JKI_lib_State_Machine.vi"("State(s) in (\"\")"=w447) -> ("States Out"=w446:string)  [unwired: 14 in]
      }
      frame "---------- UI ----------" {
        # "Do not put any code in this frame.\n(It is a separator no-op. You can make a copy of this frame to create a new UI frame)"
        n190 = call <vilib>:"Add State(s) to Queue__JKI_lib_State_Machine.vi"("State(s) in (\"\")"=w452) -> ("States Out"=w451:string)  [unwired: 14 in]
      }
      frame "UI: Initialize" {
        w457 = " " ("State History")
        # "Initialize the User Interface, here.\n(this is called automatically, by the Macro: Init)"
        n191 = Unbundle By Name(w459) -> ("Toobar.advance"=w458:refnum<vi>[])
        n192 = disable-structure shown="Disabled" {
          disable-tunnel: w458 -> [w463 _]
          frame Disabled {
            n193 = for {
              tunnel: w463 -> [w465] mode=indexing
              n194 = property class="Ctl"(reference=w465, "Visible"=FALSE) -> ()  [unwired: 1 in, 2 out]
            }
          }
          frame Enabled {
          }
        }
        n195 = local write "Tab(Msg/Status)"(enum32{"Message", "Status"}."Message" ("Tab(Msg/Status)")) -> ()
        n196 = local write "Response"(w457) -> ()
        n197 = local write "Interface-Filter"(enum16{"API-Only", "UserDef States", "All"}."UserDef States" ("Interface-Filter")) -> ()
        n198 = local write "State History"(w457) -> ()
        n199 = local write "Level"(Periodic_String_Filter_Level."normal" ("Level")) -> ()
        n200 = call <vilib>:"Add State(s) to Queue__JKI_lib_State_Machine.vi"("State(s) in (\"\")"=w462) -> ("States Out"=w461:string)  [unwired: 14 in]
      }
      frame "UI: Cursor Set" {
        # "Argument"
        # "Set and Unset Cursor Busy.\n(Usage: \"UI: Cursor Set >> Busy|Idle\")"
        n201 = case shown="\"Idle\", Default" w467 {
          tunnel: w469 -> [w474 w476]
          tunnel: [w473 w475] -> w468
          frame "Idle", Default {
            n202 = call <vilib>:"Unset Busy.vi"("error in (no error)"=w474) -> ("error out"=w473:errorcluster)  [unwired: 10 in]
          }
          frame "Busy" {
            n203 = call <vilib>:"Set Busy.vi"("error in (no error)"=w476) -> ("error out"=w475:errorcluster)  [unwired: 9 in, 1 out]
          }
        }
        n204 = call <vilib>:"Add State(s) to Queue__JKI_lib_State_Machine.vi"("State(s) in (\"\")"=w472) -> ("States Out"=w471:string)  [unwired: 14 in]
      }
      frame "UI: Front Panel State" {
        # "Argument"
        # "Set Front Panel Open or Closed\n(Usage: \"UI: Front Panel State >> Open|Close\")"
        n205 = Unbundle By Name(w480) -> ("Core.Current VI Reference"=w479:refnum<vi>)
        n206 = case shown="\"Minimize\", \"Minimized\"" w478 {
          tunnel: w482 -> [w490 w505 w516 w529 w542]
          tunnel: [w492 w506 w518 w531 w544] -> w481
          tunnel: w479 -> [w491 w503 w517 w530 w543]
          frame "Open", "Standard", Default {
            w485 = T4."Standard" ("State")
            n207 = property class="VI"(reference=w491, error in=w490) -> (reference out=w488:refnum<vi>, error out=w489:errorcluster, "FP.State"=w487:T4)
            n208 = Not Equal?(x=w487, y=w485) -> (x != y?=w486:bool)
            n209 = case shown="True" w486 {
              tunnel: [w496 w498] -> w492
              tunnel: w489 -> [w495 w498]
              tunnel: w488 -> [w494 _]
              tunnel: w485 -> [w493 _]
              frame True {
                n210 = invoke class="VI" method="FP.Open"(reference=w494, error in=w495, "Activate"=TRUE, "State"=w493) -> (error out=w496:errorcluster)  [unwired: 1 in, 4 out]
              }
              frame False {
              }
            }
          }
          frame "Close", "Closed" {
            n211 = property class="VI"(reference=w503, error in=w505) -> (reference out=w502:refnum<vi>, error out=w504:errorcluster, "FP.State"=w500:T4)
            n212 = Not Equal?(x=w500, y=T4."Closed" ("Front Panel Window:State")) -> (x != y?=w499:bool)
            n213 = case shown="True" w499 {
              tunnel: [w507 w510] -> w506
              tunnel: w504 -> [w507 w509]
              tunnel: w502 -> [_ w508]
              frame False {
              }
              frame True {
                n214 = invoke class="VI" method="FP.Close"(reference=w508, error in=w509) -> (error out=w510:errorcluster)  [unwired: 1 in, 2 out]
              }
            }
          }
          frame "Hidden", "Hide" {
            w511 = T4."Hidden" ("State")
            n215 = property class="VI"(reference=w517, error in=w516) -> (reference out=w514:refnum<vi>, error out=w515:errorcluster, "FP.State"=w513:T4)
            n216 = Not Equal?(x=w513, y=w511) -> (x != y?=w512:bool)
            n217 = case shown="True" w512 {
              tunnel: [w522 w523] -> w518
              tunnel: w515 -> [w521 w523]
              tunnel: w514 -> [w520 _]
              tunnel: w511 -> [w519 _]
              frame True {
                n218 = invoke class="VI" method="FP.Open"(reference=w520, error in=w521, "State"=w519) -> (error out=w522:errorcluster)  [unwired: 2 in, 4 out]
              }
              frame False {
              }
            }
          }
          frame "Minimize", "Minimized" {
            w524 = T4."Minimized" ("State")
            n219 = property class="VI"(reference=w530, error in=w529) -> (reference out=w527:refnum<vi>, error out=w528:errorcluster, "FP.State"=w526:T4)
            n220 = Not Equal?(x=w526, y=w524) -> (x != y?=w525:bool)
            n221 = case shown="True" w525 {
              tunnel: [w535 w536] -> w531
              tunnel: w528 -> [w534 w536]
              tunnel: w527 -> [w533 _]
              tunnel: w524 -> [w532 _]
              frame True {
                n222 = invoke class="VI" method="FP.Open"(reference=w533, error in=w534, "State"=w532) -> (error out=w535:errorcluster)  [unwired: 2 in, 4 out]
              }
              frame False {
              }
            }
          }
          frame "Maximize", "Maximized" {
            w537 = T4."Maximized" ("State")
            n223 = property class="VI"(reference=w543, error in=w542) -> (reference out=w540:refnum<vi>, error out=w541:errorcluster, "FP.State"=w539:T4)
            n224 = Not Equal?(x=w539, y=w537) -> (x != y?=w538:bool)
            n225 = case shown="True" w538 {
              tunnel: [w548 w549] -> w544
              tunnel: w541 -> [w547 w549]
              tunnel: w540 -> [w546 _]
              tunnel: w537 -> [w545 _]
              frame True {
                n226 = invoke class="VI" method="FP.Open"(reference=w546, error in=w547, "State"=w545) -> (error out=w548:errorcluster)  [unwired: 2 in, 4 out]
              }
              frame False {
              }
            }
          }
        }
        n227 = call <vilib>:"Add State(s) to Queue__JKI_lib_State_Machine.vi"("State(s) in (\"\")"=w484) -> ("States Out"=w483:string)  [unwired: 14 in]
      }
      frame "UI: Autoset Arguments" {
        n228 = call "CSM - Revert Arguments-Safe String.vi"("Safe Argument String"=w563) -> ("Origin Argument String"=w550:string)  [unwired: 8 in]
        n229 = control-ref of="CSM"() -> (w558:refnum<vi>)
        n230 = call "Remove Comments from Single-line.vi"("single-line text"=w550) -> ("single-line text without comments"=w562:string)  [unwired: 2 in]
        n231 = property on="Property Node" class="CmbBox"(reference=w558) -> (reference out=w556:refnum<vi>, "Strings[]"=w557:string[])  [unwired: 1 in, 1 out]
        n232 = call "Split Single-line Message.vi"("single-line text"=w562) -> ("state"=w560:string, "args"=w559:string, "source/target"=w552:string)  [unwired: 6 in, 1 out]
        n233 = case shown="\"<interrupt>\", \"<status>\"" w552 {
          selector: w552 -> [w566 _]
          tunnel: [w566 w568] -> w551
          tunnel: w550 -> [_ w569]
          frame Default {
            n234 = property on="Tab(Msg/Status)" class="TabCtl (strict)"("Val(Sgnl)"=enum32{"Message", "Status"}."Message" ("Tab(Msg/Status)")) -> ()  [unwired: 2 in, 2 out]
          }
          frame "<interrupt>", "<status>" {
            n235 = Match Pattern(string=w569, regular expression="//") -> (after substring=w568:string)  [unwired: 1 in, 3 out]
            n236 = property on="Tab(Msg/Status)" class="TabCtl (strict)"("Val(Sgnl)"=enum32{"Message", "Status"}."Status" ("Tab(Msg/Status)")) -> ()  [unwired: 2 in, 2 out]
          }
        }
        n237 = local write "MsgString"(w560) -> ()
        n238 = local write "Arguments"(w559) -> ()
        n239 = Search 1D Array(1D array=w557, element=w551) -> (index of element=w555:i32)  [unwired: 1 in]
        n240 = Greater Or Equal To 0?(x=w555) -> (x >= 0?=w554:bool)
        n241 = case shown="True" w554 {
          tunnel: w556 -> [_ w573]
          tunnel: w551 -> [_ w572]
          frame False {
          }
          frame True {
            n242 = property on="Property Node" class="CmbBox"(reference=w573, "Value"=w572) -> ()  [unwired: 1 in, 2 out]
          }
        }
      }
      frame "UI: Refresh History List" {
        n243 = Unbundle By Name(w580) -> ("MessageList"=w577:string[])
        n244 = property on="History" class="LstBox (strict)"() -> ("Item Names"=w578:string[], "Value"=w579:i32)  [unwired: 2 in, 2 out]
        n245 = Index Array(array=w578, index=w579) -> (element=w574:string)
        n246 = Search 1D Array(1D array=w577, element=w574) -> (index of element=w575:i32)  [unwired: 1 in]
        n247 = property on="History" class="LstBox (strict)"("Item Names"=w577, "Value"=w575) -> ()  [unwired: 2 in, 2 out]
      }
      frame "UI: Refresh CSM List" {
        n248 = control-ref of="CSM"() -> (w593:refnum<vi>)
        n249 = property on="Property Node" class="CmbBox"(reference=w593) -> (reference out=w585:refnum<vi>, "Value"=w589:string)  [unwired: 1 in, 1 out]
        n250 = call "CSM - List Modules.vi"("Scope (Normal)"="Scope") -> ("error out"=w592:errorcluster, "Module Names"=w587:string[])  [unwired: 9 in]
        n251 = Search 1D Array(1D array=w587, element=w589) -> (index of element=w591:i32)  [unwired: 1 in]
        n252 = Greater Or Equal To 0?(x=w591) -> (x >= 0?=w590:bool)
        n253 = Index Array(array=w587) -> (element=w588:string)  [unwired: 1 in]
        n254 = Select(t=w589, s=w590, f=w588) -> (s? t:f=w586:string)
        n255 = property on="Property Node" class="CmbBox"(reference=w585, "Strings[]"=w587, "Value"=w586) -> ()  [unwired: 1 in, 2 out]
        n256 = call <vilib>:"Simple Error Handler.vi"("error in (no error)"=w592) -> ()  [unwired: 4 in, 5 out]
      }
      frame "UI: Refresh UI" {
      }
      frame "---------- Macro ----------" {
        # "Do not put any code in this frame.\n(It is a separator no-op. You can make a copy of this frame to create a new Macro frame)"
        n257 = call <vilib>:"Add State(s) to Queue__JKI_lib_State_Machine.vi"("State(s) in (\"\")"=w605) -> ("States Out"=w604:string)  [unwired: 14 in]
      }
      frame "Macro: Initialize" {
        # "Initialization Macro\n(This is called once, when the VI starts)"
        n258 = call <vilib>:"Add State(s) to Queue__JKI_lib_State_Machine.vi"("State(s) in Front (\"\")"="Data: Initialize\nData: Initialize References\nInitialize Core Data\nEvents: Register\nUI: Initialize\nData: Load Arguments Config File\nUI: Front Panel State >> Open\nUI: Refresh CSM List\nUI: Refresh History List\nUI: Refresh UI\nAction: Refresh API List\nAction: Change Btn States", "State(s) in (\"\")"=w611) -> ("States Out"=w610:string)  [unwired: 13 in]
      }
      frame "Macro: Exit" {
        # "Exit Macro\n(This is called once, when the VI exits)"
        n259 = Unbundle By Name(w619) -> ("Core.Close Panel on Exit?"=w618:bool)
        n260 = Select(t="UI: Front Panel State >> Close", s=w618, f="") -> (s? t:f=w615:string)
        n261 = call <vilib>:"Add State(s) to Queue__JKI_lib_State_Machine.vi"("State(s) in (\"\")"=w615, "State(s) at Back (\"\")"="Data: Save Arguments Config File\nData: Cleanup\nEvents: Unregister\nExit") -> ("States Out"=w613:string)  [unwired: 13 in]
        n262 = call <vilib>:"Add State(s) to Queue__JKI_lib_State_Machine.vi"("State(s) in Front (\"\")"=w613, "State(s) in (\"\")"=w622) -> ("States Out"=w621:string)  [unwired: 13 in]
      }
      frame "---------- Action ----------" {
        # "Template Separator\n(You can make a copy of, or modify, this frame)"
        n263 = call <vilib>:"Add State(s) to Queue__JKI_lib_State_Machine.vi"("State(s) in (\"\")"=w627) -> ("States Out"=w626:string)  [unwired: 14 in]
      }
      frame "Action: Send CSM Message" {
        n264 = local read "CSM"() -> (w633:string)
        n265 = Multiply(x=1000, y="Timeout(s)") -> (x*y=w630:i32)
        n266 = case shown="Default" "MsgString" {
          selector: "MsgString" -> [_ w647]
          tunnel: "Arguments" -> [_ w646]
          tunnel: [_ w652] -> w634
          tunnel: w633 -> [_ w645]
          tunnel: [_ w644] -> w632
          tunnel: w630 -> [_ w651]
          frame "" {
          }
          frame Default {
            n267 = call "CSM - Send Message and Wait for Reply.vi"("Response Timeout (-2 Using Global Settings)"=w651, "Current Module (\"\" to Generate an ID)"="Tool-Testpnl" ("Current Module(\"\" to generate an ID)"), "Target Module"=w645, "Arguments (\"\")"=w646, "State"=w647) -> ("error out"=w652:errorcluster, "Response"=w654:string)  [unwired: 4 in, 1 out]
            n268 = call-poly "Build Message with Arguments++.vi"("State With Arguments"=w647, "Arguments (\"\")"=w646, "Target Module (\"\")"=w645) -> ("CSM Message String"=w649:string)  [unwired: 12 in]
            n269 = case shown="True" "Revert Safe String" {
              tunnel: w654 -> [w655 w657]
              tunnel: [w655 w656] -> w641
              frame False {
              }
              frame True {
                n270 = call "CSM - Revert Arguments-Safe String.vi"("Safe Argument String"=w657) -> ("Origin Argument String"=w656:string)  [unwired: 8 in]
              }
            }
            "Response" <- w641
            n271 = call "CSM - Make String Arguments Safe.vi"("Argument String"=w649) -> ("Safe Argument String"=w648:string)  [unwired: 8 in]
            n272 = call <vilib>:"Build State String with Arguments__JKI_lib_State_Machine.vi"("Arguments (\"\")"=w648, "State"="Data: Update Message List" ("State(s) in Front (\"\")")) -> ("State with Arguments"=w643:string)  [unwired: 4 in]
            n273 = call <vilib>:"Add State(s) to Queue__JKI_lib_State_Machine.vi"("State(s) in (\"\")"=w643, "State(s) at Back (\"\")"="UI: Refresh History List\nData: Save Arguments Config File" ("State(s) in Front (\"\")")) -> ("States Out"=w644:string)  [unwired: 13 in]
          }
        }
        n274 = call <vilib>:"Add State(s) to Queue__JKI_lib_State_Machine.vi"("State(s) in (\"\")"=w639, "State(s) at Back (\"\")"=w632) -> ("States Out"=w638:string)  [unwired: 13 in]
      }
      frame "Action: Post CSM Message" {
        # "Your code here.\n(You can make a copy of, or modify, this frame)"
        n275 = local read "MsgString"() -> (w659:string)
        n276 = local read "Arguments"() -> (w660:string)
        n277 = local read "CSM"() -> (w662:string)
        n278 = case shown="Default" w659 {
          selector: w659 -> [_ w672]
          tunnel: w660 -> [_ w671]
          tunnel: [_ w676] -> w663
          tunnel: w662 -> [_ w670]
          tunnel: [_ w669] -> w661
          frame "" {
          }
          frame Default {
            n279 = call "CSM - Post Message.vi"("Current Module (\"\" to Generate an ID)"="Tool-Testpnl" ("Current Module(\"\" to generate an ID)"), "Target Module"=w670, "Arguments (\"\")"=w671, "State"=w672) -> ("error out"=w676:errorcluster)  [unwired: 7 in]
            n280 = call-poly "Build Message with Arguments++.vi"("State With Arguments"=w672, "Arguments (\"\")"=w671, "Target Module (\"\")"=w670) -> ("CSM Message String"=w674:string)  [unwired: 12 in]
            n281 = call "CSM - Make String Arguments Safe.vi"("Argument String"=w674) -> ("Safe Argument String"=w673:string)  [unwired: 8 in]
            n282 = call <vilib>:"Build State String with Arguments__JKI_lib_State_Machine.vi"("Arguments (\"\")"=w673, "State"="Data: Update Message List" ("State(s) in Front (\"\")")) -> ("State with Arguments"=w668:string)  [unwired: 4 in]
            n283 = call <vilib>:"Add State(s) to Queue__JKI_lib_State_Machine.vi"("State(s) in (\"\")"=w668, "State(s) at Back (\"\")"="UI: Refresh History List\nData: Save Arguments Config File" ("State(s) in Front (\"\")")) -> ("States Out"=w669:string)  [unwired: 13 in]
          }
        }
        n284 = call <vilib>:"Add State(s) to Queue__JKI_lib_State_Machine.vi"("State(s) in (\"\")"=w666, "State(s) at Back (\"\")"=w661) -> ("States Out"=w665:string)  [unwired: 13 in]
      }
      frame "Action: Broadcast Status" {
        # "Your code here.\n(You can make a copy of, or modify, this frame)"
        n285 = local read "MsgString"() -> (w679:string)
        n286 = local read "Arguments"() -> (w680:string)
        n287 = local read "CSM"() -> (w682:string)
        n288 = case shown="Default" w679 {
          selector: w679 -> [_ w689]
          tunnel: w680 -> [_ w688]
          tunnel: [_ w690] -> w683
          tunnel: w682 -> [_ w687]
          tunnel: [_ w695] -> w681
          frame "" {
          }
          frame Default {
            (unwired) "Tool-Testpnl" ("Current Module(\"\" to generate an ID)")
            n289 = call "CSM - Request CSM to Broadcast Status Change.vi"("Module Name"=w687, "Arguments (\"\")"=w688, "Status"=w689) -> ("error out"=w690:errorcluster)  [unwired: 8 in]
            n290 = call-poly "Build Message with Arguments++.vi"("State With Arguments"=w689, "Arguments (\"\")"=w688) -> ("CSM Message String"=w697:string)  [unwired: 13 in]
            n291 = Concatenate Strings(w697, "//" ("string"), w687) -> (w692:string)
            n292 = call "CSM - Make String Arguments Safe.vi"("Argument String"=w692) -> ("Safe Argument String"=w696:string)  [unwired: 8 in]
            n293 = call <vilib>:"Build State String with Arguments__JKI_lib_State_Machine.vi"("Arguments (\"\")"=w696, "State"="Data: Update Message List" ("State(s) in Front (\"\")")) -> ("State with Arguments"=w694:string)  [unwired: 4 in]
            n294 = call <vilib>:"Add State(s) to Queue__JKI_lib_State_Machine.vi"("State(s) in (\"\")"=w694, "State(s) at Back (\"\")"="UI: Refresh History List\nData: Save Arguments Config File" ("State(s) in Front (\"\")")) -> ("States Out"=w695:string)  [unwired: 13 in]
          }
        }
        n295 = call <vilib>:"Add State(s) to Queue__JKI_lib_State_Machine.vi"("State(s) in (\"\")"=w686, "State(s) at Back (\"\")"=w681) -> ("States Out"=w685:string)  [unwired: 13 in]
      }
      frame "Action: Change Btn States" {
        n296 = local read "CSM"() -> (w700:string)
        n297 = case shown="Default" w700 {
          selector: w700 -> [_ w719]
          tunnel: w699 -> [_ w718]
          frame "" {
          }
          frame Default {
            n298 = call "CSM - Module VI Reference.vi"("Response Timeout (-2 Using Global Settings)"=1000 ("Response Timeout(5000 ms)"), "Current Module (\"\" to Generate an ID)"=w718, "error in (no error)"=errorcluster {"status"=FALSE, "code"=0, "source"=""}, "CSM Name"=w719) -> ("error out"=w714:errorcluster, "CSM Module VIRef"=w715:refnum<vi>)  [unwired: 6 in]
            n299 = property class="VI"(reference=w715, error in=w714) -> (reference out=w708:refnum<vi>, "IsInPackedLibrary"=→"inlvlibp":bool, "Diagram"=w707:refnum<vi>)  [unwired: 1 out]
            n300 = Not A Number/Path/Refnum?(number/path/refnum=w707) -> (NaN/Path/Refnum?=w711:bool)
            n301 = Select(t=2, s=w711, f=0) -> (s? t:f=w712:i32)
            n302 = Close Reference(reference=w707) -> (error out=w706:errorcluster)  [unwired: 1 in]
            n303 = call <vilib>:"Clear Errors.vi"("error in (no error)"=w706) -> ("error out"=w705:errorcluster)  [unwired: 5 in, 1 out]
            n304 = property on="Toolbar.Open BD" class="Bool"("DisabledEnum"=w712) -> ()  [unwired: 2 in, 2 out]
            n305 = Close Reference(reference=w708, error in (no error)=w705) -> ()  [unwired: 1 out]
          }
        }
      }
      frame "Action: Refresh API List" {
        n306 = local read "Tab(Msg/Status)"() -> (w724:enum32{"Message", "Status"})
        n307 = local read "CSM"() -> (w726:string)
        n308 = in-place {
          in-place-border: w726 -> [w737]
          in-place-border: [w736] -> w729
          n309 = in-place-cluster #1(w728) -> ("CSM Check History"=w735:string[])
          n310 = Search 1D Array(1D array=w735, element=w737) -> (index of element=w738:i32)  [unwired: 1 in]
          n311 = Less Than 0?(x=w738) -> (x < 0?=w736:bool)
          n312 = case shown="True" w736 {
            tunnel: w735 -> [w739 w742]
            tunnel: w737 -> [_ w741]
            tunnel: [w739 w740] -> w734
            frame False {
            }
            frame True {
              n313 = Build Array (concatenate)(w742, w741) -> (w740:string[])
            }
          }
          n314 = in-place-cluster #1("CSM Check History"=w734) -> (w727:T10)
        }
        n315 = call "CSM - Check If Module Exists.vi"("CSM Name"=w726) -> ("error out"=w721:errorcluster, "Exist?"=w722:bool, "CSM Name (Dup)"=w732:string)  [unwired: 8 in]
        n316 = Not(x=w721) -> (.not. x?=w720:bool)
        n317 = And(x=w722, y=w720) -> (x .and. y?=w723:bool)
        n318 = case shown="True" w723 {
          tunnel: w732 -> [_ w763]
          tunnel: w731 -> [_ w762]
          tunnel: [_ w764] -> w730
          tunnel: w729 -> [_ w761]
          tunnel: w726 -> [_ w760]
          tunnel: w724 -> [w743 w756]
          frame False {
            n319 = case shown="\"Message\", Default" w743 {
              tunnel: [T7."Enabled" ("Disabled") T7."Disabled and Grayed Out" ("Disabled")] -> w744
              frame "Message", Default {
              }
              frame "Status" {
              }
            }
            n320 = property on="Revert Safe String" class="Bool (strict)"("DisabledEnum"=w744) -> ()  [unwired: 2 in, 2 out]
            n321 = property on="Arguments" class="Str"("DisabledEnum"=w744) -> ()  [unwired: 2 in, 2 out]
            n322 = property on="Response" class="Str"("DisabledEnum"=w744) -> ()  [unwired: 2 in, 2 out]
          }
          frame True {
            n323 = case shown="\"Status\"" w756 {
              tunnel: [w770 w784] -> w764
              tunnel: w763 -> [w772 w783]
              tunnel: w762 -> [w771 w782]
              tunnel: w761 -> [w769 w781]
              tunnel: [w766 w779] -> w753
              tunnel: [T7."Disabled and Grayed Out" ("Disabled") T7."Enabled" ("Disabled")] -> w751
              frame "Status" {
                n324 = call "Read CSM Status with lvcsm Support.vi"("Current Module (\"\" to Generate an ID)"=w771, "Force? (F)"=w769, "CSM Name"=w772) -> ("error out"=w770:errorcluster, "CSMAPI List"=w768:string[])  [unwired: 7 in]
                n325 = for {
                  tunnel: w768 -> [w776] mode=indexing
                  tunnel: [w773] -> w767 mode=indexing
                  n326 = Match Pattern(string=w776, regular expression="@") -> (before substring=w774:string)  [unwired: 1 in, 3 out]
                  n327 = call "Trim Single-line Text.vi"("single-line text"=w774) -> ("trimed text"=w773:string)  [unwired: 2 in]
                }
                n328 = call "Remove Duplicates From StrArray.vi"("StrArray In"=w767) -> ("StrArray"=w766:string[])  [unwired: 9 in, 1 out]
              }
              frame "Message" {
                n329 = call "Read CSM States with lvcsm Support.vi"("Current Module (\"\" to Generate an ID)"=w782, "Force? (F)"=w781, "CSM Name"=w783) -> ("error out"=w784:errorcluster, "CSMAPI List"=w780:string[])  [unwired: 7 in]
                n330 = call "filter CSM States.vi"("Interface-Filter"="Interface-Filter", "Array"=w780) -> ("filtered array"=w779:string[])  [unwired: 9 in]
              }
            }
            n331 = call "CSM - Module VI Reference.vi"("CSM Name"=w760) -> ("error out"=w758:errorcluster, "CSM Module VIRef"=w759:refnum<vi>)  [unwired: 9 in]
            n332 = property class="VI"(reference=w759, error in=w758) -> ("Exec.PostExecutionProbes"=w757:bool)  [unwired: 2 out]
            n333 = local write "RetainWireValues"(w757) -> ()
            n334 = property on="Revert Safe String" class="Bool (strict)"("DisabledEnum"=w751) -> ()  [unwired: 2 in, 2 out]
            n335 = property on="Arguments" class="Str"("DisabledEnum"=w751) -> ()  [unwired: 2 in, 2 out]
            n336 = property on="Response" class="Str"("DisabledEnum"=w751) -> ()  [unwired: 2 in, 2 out]
            n337 = property on="Message/Status" class="CmbBox"("Strings[]"=w753) -> ("Value"=w754:string)  [unwired: 2 in, 2 out]
            n338 = Search 1D Array(1D array=w753, element=w754) -> (index of element=w755:i32)  [unwired: 1 in]
            n339 = Index Array(array=w753) -> (element=w748:string)  [unwired: 1 in]
            n340 = Greater Or Equal To 0?(x=w755) -> (x >= 0?=w749:bool)
            n341 = Empty String/Path?(string/path=w748) -> (empty?=w747:bool)
            n342 = Or(x=w749, y=w747) -> (x .or. y?=w750:bool)
            n343 = Select(t=w754, s=w750, f=w748) -> (s? t:f=w752:string)
            n344 = property on="Message/Status" class="CmbBox"("Value"=w752) -> ()  [unwired: 2 in, 2 out]
          }
        }
      }
      frame "No Peroidic Log over 1s" {
        n345 = call "CSM - Generate User Global Log.vi"("Place (\"\" to Use VI's Name)"=w785, "Log"="No Peroidic Log over 1s.") -> ()  [unwired: 9 in, 1 out]
      }
    }
  }
  n346 = while {
    shift-right: [w823] -> w13
    shift-left: w10 -> [w820]
    shift-right: [w813] -> w12
    shift-left: w11 -> [w824]
    shift-right: [w806] -> w5
    shift-left: w4 -> [w806]
    stop <- w810 stop-if-true
    n347 = Get Queue Status(queue=w824, error in (no error)=w820) -> (queue out=w822:refnum<queue>, error out=w821:errorcluster, # elements in queue=w809:i32)  [unwired: 1 in, 5 out]
    "LogInQ" <- w809
    n348 = call "Auto Processing Level.vi"("#Left In Q"=w809) -> ("Level"=w800:T3)  [unwired: 8 in, 2 out]
    n349 = feedback #2(Periodic_String_Filter_Level."normal" ("Level")) -> (w803:T3)
    n350 = feedback-in #2(w800) -> ()
    n351 = Not Equal?(x=w800, y=w803) -> (x != y?=w801:bool)
    n352 = case shown="True" w801 {
      tunnel: w800 -> [_ w842]
      frame False {
      }
      frame True {
        n353 = local write "Level"(w842) -> ()
      }
    }
    n354 = Dequeue Element(queue=w822, timeout in ms (-1)=100, error in (no error)=w821) -> (queue out=w813:refnum<queue>, element=w819:T13, timed out?=w804:bool, error out=w823:errorcluster)
    n355 = Not(x=w804) -> (.not. x?=w805:bool)
    n356 = call "Occurrence Speed Counter.vi"("Period (0.1s)"=1.0 ("period(0.1s)"), "Occured? (T)"=w805) -> ("Speed (#/s)"=w798:dbl)  [unwired: 7 in, 2 out]
    "handling Speed(#/s)" <- w798
    n357 = Equal To 0?(x=w798) -> (x = 0?=w797:bool)
    n358 = Unbundle By Name("Settings") -> ("Check Peroid(s)"=w791:dbl)
    n359 = Add(x=w791, y=w791) -> (x+y=w792:dbl)
    n360 = call "Debounced Signal.vi"("Debounce Period (5s)"=w792, "Signal"=w797) -> ("Since Last Change (S)"=w793:dbl, "Signal (Safe)"=w795:bool)  [unwired: 8 in]
    n361 = call "Rising Edge.vi"("Signal"=w795) -> ("Rising Edge"=w794:bool)
    n362 = case shown="True" w794 {
      tunnel: w793 -> [_ w826]
      frame False {
      }
      frame True {
        n363 = Format Into String(format string="No Log for %.0fs", w826) -> (resulting string=w827:string)  [unwired: 2 in, 1 out]
        n364 = call "CSM - Generate User Global Log.vi"("Place (\"\" to Use VI's Name)"="CSM Debug Console", "Log"=w827) -> ()  [unwired: 9 in, 1 out]
      }
    }
    n365 = feedback #3("" ("String Cache")) -> (w815:string)
    n366 = case shown="False" w804 {
      tunnel: w819 -> [w835 _]
      tunnel: [w837 w840] -> w816
      tunnel: w815 -> [_ w840]
      tunnel: w806 -> [w834 _]
      tunnel: "Settings" -> [w829 _]
      frame False {
        n367 = Unbundle By Name(w835) -> ("LogType"=w836:T15)
        n368 = case shown="\"Module Created\", \"Module Destroyed\"" w836 {
          tunnel: w834 -> [_ w839]
          frame "User Log", Default {
          }
          frame "Module Created", "Module Destroyed" {
            n369 = Generate User Event(user event=w839, event data cluster="UI: Refresh CSM List" ("State(s) in Front (\"\")")) -> ()  [unwired: 2 in, 2 out]
          }
        }
        n370 = Not(x="Periodic") -> (.not. x?=w830:bool)
        n371 = call "Global Log History Cacher.vi"("Global Log Data"=w835, "Reset?"=w830, "With Periodic Info? (T)"="Periodic Info", "Settings"=w829, "Level (Normal)"="Level") -> ("String Cache"=w837:string)  [unwired: 10 in]
      }
      frame True {
      }
    }
    n372 = feedback-in #3(w816) -> ()
    n373 = Compound Arithmetic op=OR(w823, "internal-stop") -> (w811:bool)
    n374 = call "Exit With Empty Queue Check.vi"("Queue"=w813, "Timeout (5s)"=1.0 ("timeout(5s)"), "Stop"=w811) -> ("Exit"=w810:bool)  [unwired: 7 in, 1 out]
    n375 = call "Check Timeout.vi"() -> ("Timeout"=w817:bool)  [unwired: 8 in]
    n376 = Or(x=w810, y=w817) -> (x .or. y?=w812:bool)
    n377 = case shown="True" w812 {
      tunnel: w816 -> [_ w841]
      frame False {
      }
      frame True {
        "State History" <- w841
      }
    }
  }
  n378 = Merge Errors(w8, w13) -> (w9:errorcluster)
  n379 = call "CSM - Destroy Global Log Queue.vi"("Error In"=w9, "Global Log Queue"=w12) -> ("error out"=w6:errorcluster)  [unwired: 9 in]
  n380 = Destroy User Event(user event=w5, error in=w6) -> (error out=w1:errorcluster)
  n381 = control-ref of="Current VI Reference"() -> (w2:refnum<vi>)
  n382 = call "Close FP if in LabVIEW Dir.vi"("VI Refnum"=w2, "Error in"=w1) -> ("Error out"=w3:errorcluster)  [unwired: 9 in]
  n383 = call <vilib>:"Clear Errors.vi"("error in (no error)"=w3) -> ()  [unwired: 5 in, 2 out]
